vi "Autonomous Independent.vi"   [LabVIEW 2016]
doc: "This VI is called when autonomous begins, and will automatically be terminated when autonomous ends. You can carry out timed or sensor driven robot movement independently without needing to return to the caller."
uses:
  Robot Global Data.vi
  <vilib>/Rock Robotics/Network Tables/NT Read String.vi
  <vilib>/Rock Robotics/WPI/Utilities/WPI_GetSetVariantRefNum.vi
  <vilib>/Rock Robotics/WPI/RobotDrive/WPI_RobotDriveArcadeDrive_Standard(NoSaturation).vi
panel:
  # "Be sure to right-click and choose Data Operations>>Make Current Value default if you want to save the array values with the VI"
types:
  T1 = typedef "WPI_RobotDriveDevRef.ctl" = cluster{"DevStatus":errorcluster, "Motors[]":T2[], "Square Inputs":bool, "Max Output":dbl}
  T2 = typedef "WPI_MotorControlDeviceRef.ctl" = cluster{"DeviceStatus":errorcluster, "Type":T3, "PWM":cluster{"PWM Channel":T4, "DeadBand":T5}, "CAN":cluster{"Device Number":u8, "SetOutput VI Ref":variant, "GetOutput VI Ref":variant, "Enable VI Ref":variant, "Disable VI Ref":variant, "Data":variant}, "Invert":bool}
  T3 = typedef "WPI_MotorControlType.ctl" = enum16{"PWM", "CAN"}
  T4 = typedef "FPGA_DIOPWMChannel.ctl" = enum8{"PWM 0", "PWM 1", "PWM 2", "PWM 3", "PWM 4", "PWM 5", "PWM 6", "PWM 7", "PWM 8", "PWM 9", "PWM MXP 0", "PWM MXP 1", "PWM MXP 2", "PWM MXP 3", "PWM MXP 4", "PWM MXP 5", "PWM MXP 6", "PWM MXP 7", "PWM MXP 8", "PWM MXP 9", "Invalid"}
  T5 = typedef "WPI_PWMDeadband.ctl" = cluster{"Name":string, "maxPositivePwm":i32, "minPositivePwm":i32, "centerPwm":i32, "maxNegativePwm":i32, "minNegativePwm":i32, "angularRange":u16}
  T6 = typedef "WPI_GyroDevRef.ctl" = cluster{"DevStatus":errorcluster, "Analog Channel":T7, "Offset":dbl, "Gain (VoltsPerDegree/Second)":dbl, "Gyro Type":enum16{"Analog", "XRS450"}, "Handle":i32, "SPI Bus":T8, "Device Found":bool, "Sample Rate":dbl, "Calibrate On Open":bool}
  T7 = typedef "FPGA_AIChannel.ctl" = enum8{"AI 0", "AI 1", "AI 2", "AI 3", "AI MXP 0", "AI MXP 1", "AI MXP 2", "AI MXP 3", "Invalid"}
  T8 = typedef "spi_bus.ctl" = enum16{"SPI On-Board, CS0", "SPI On-Board, CS1", "SPI On-Board, CS2", "SPI On-Board, CS3", "SPI MXP", "Invalid"}
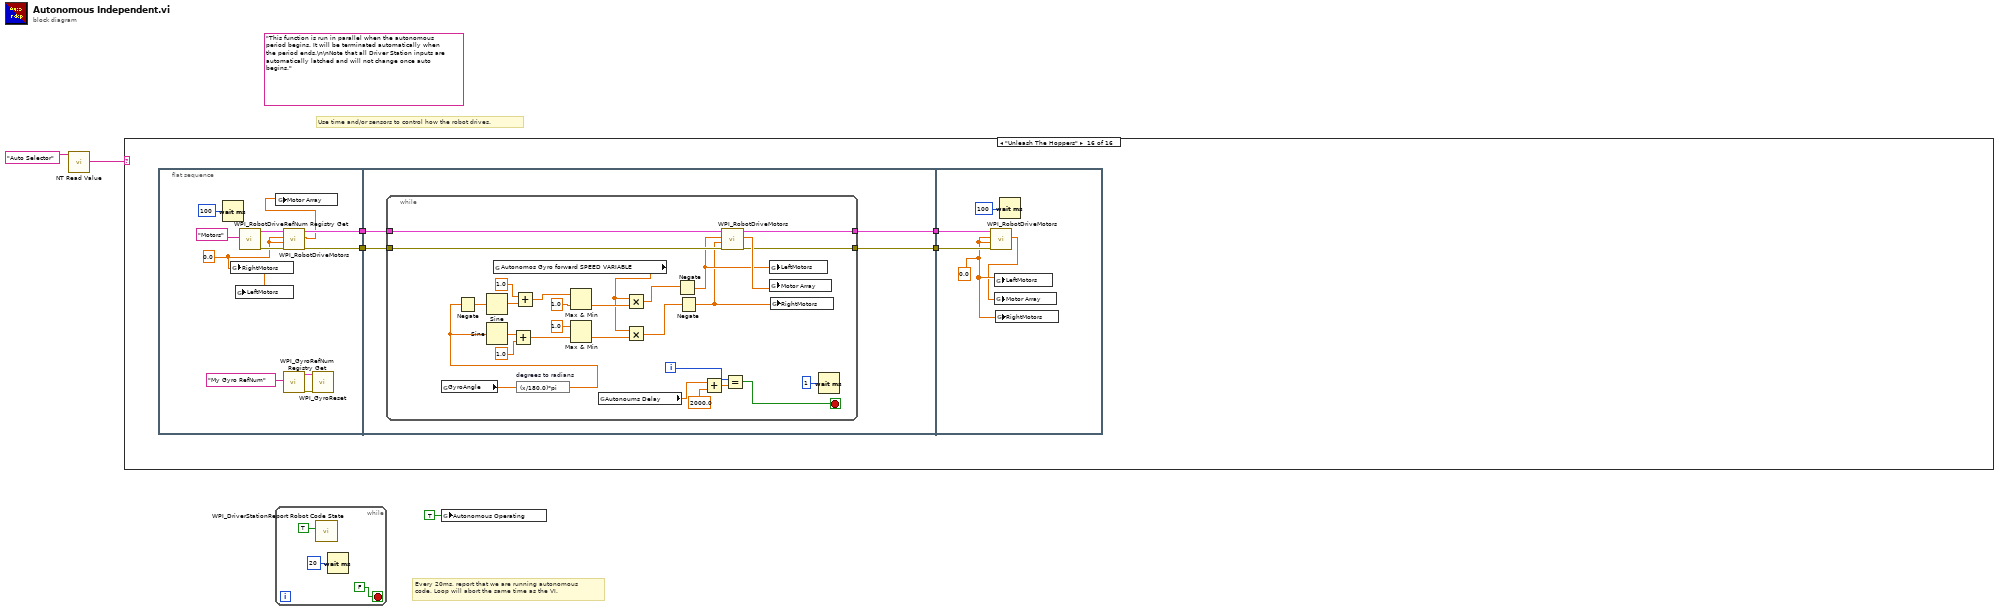
[diagram p0: block diagram]
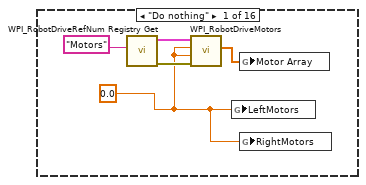
[diagram p2: hidden frame]
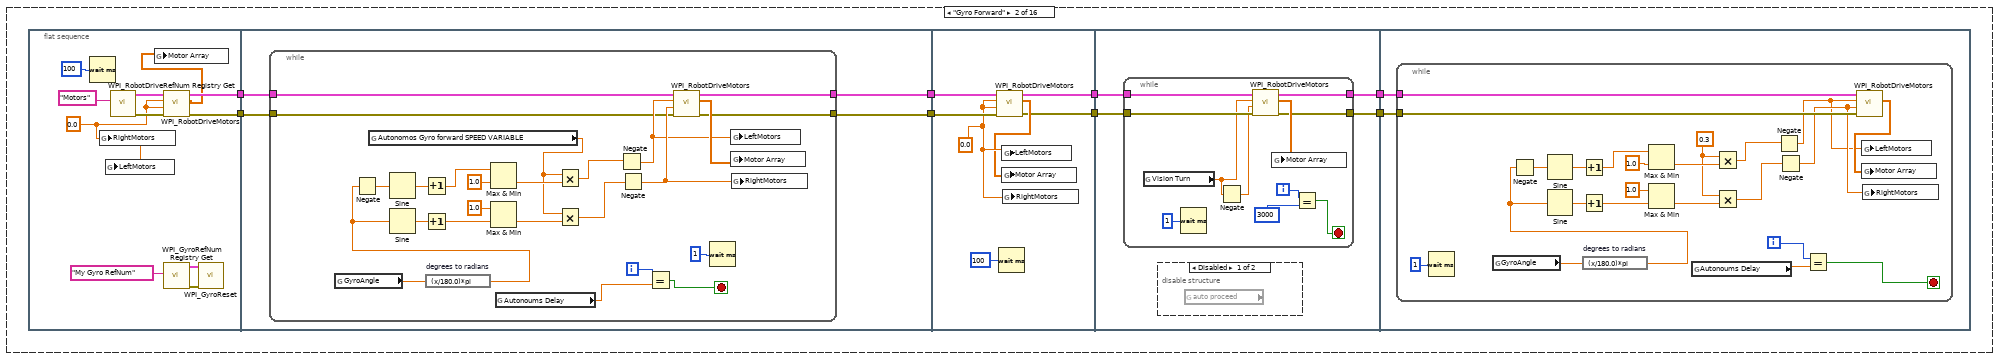
[diagram p3: hidden frame]
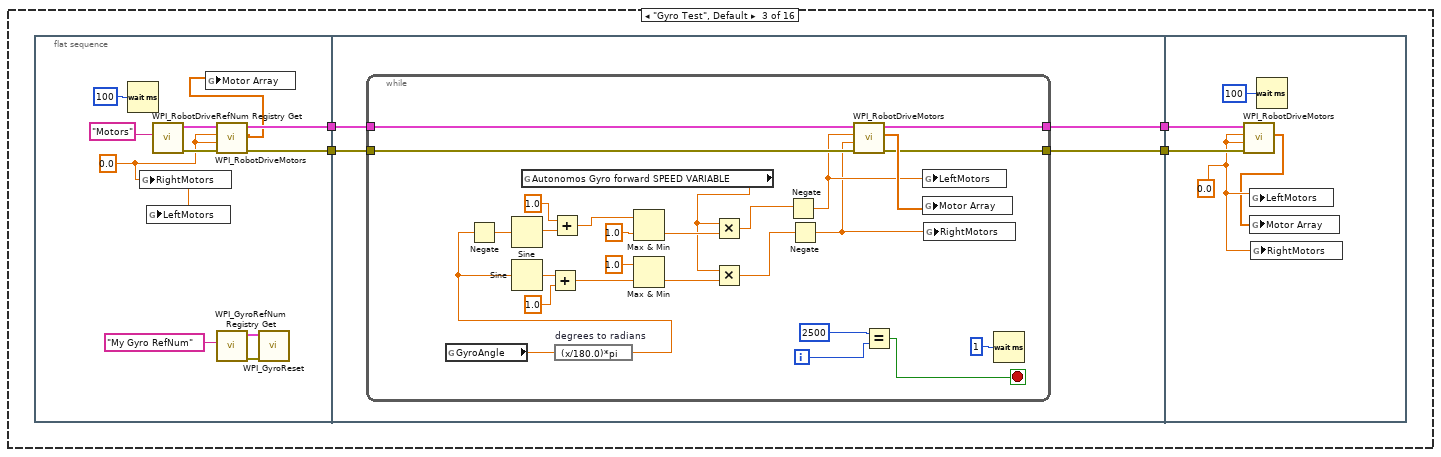
[diagram p5: hidden frame]
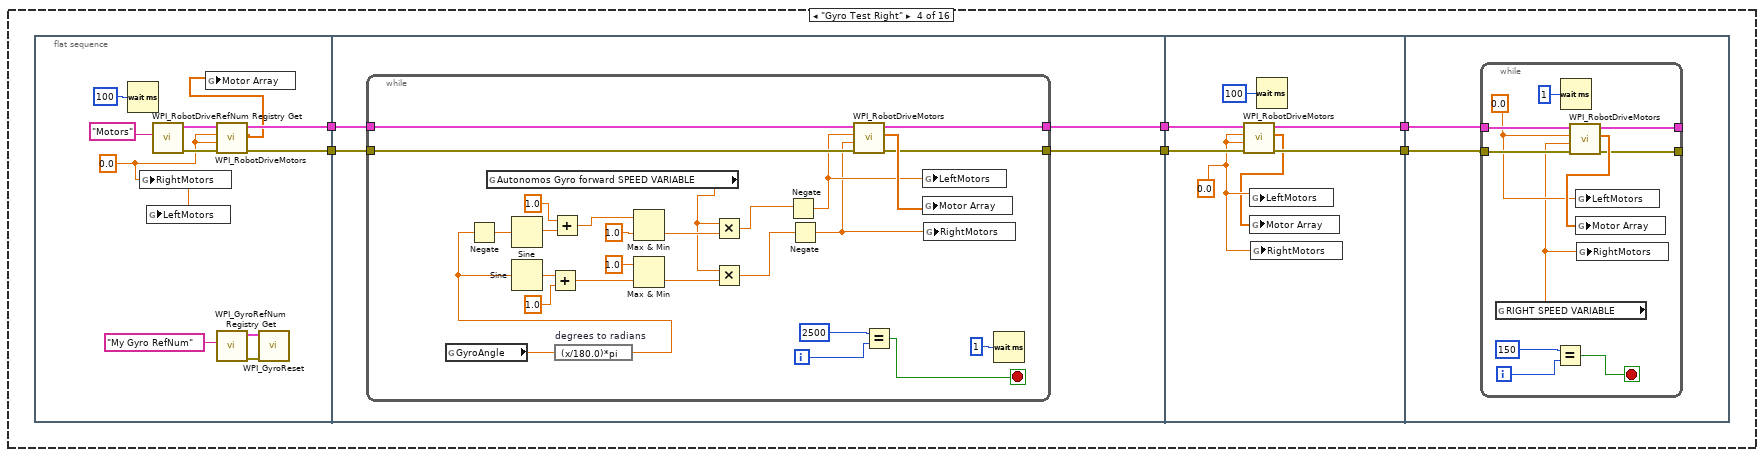
[diagram p6: hidden frame]
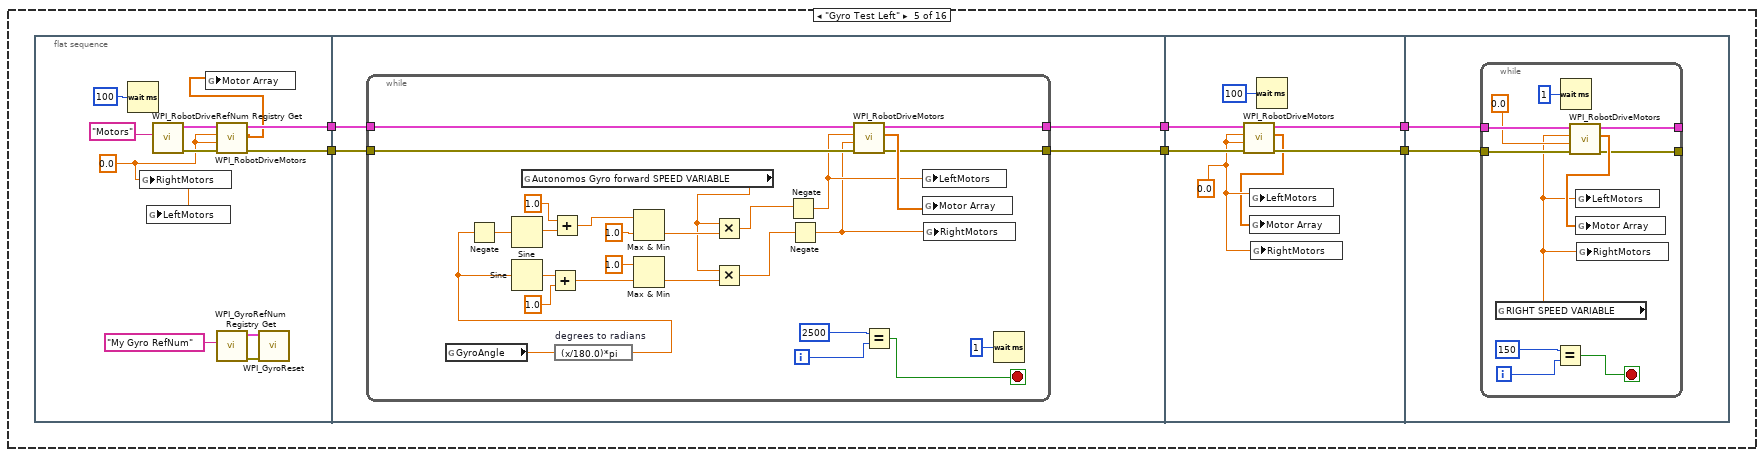
[diagram p7: hidden frame]
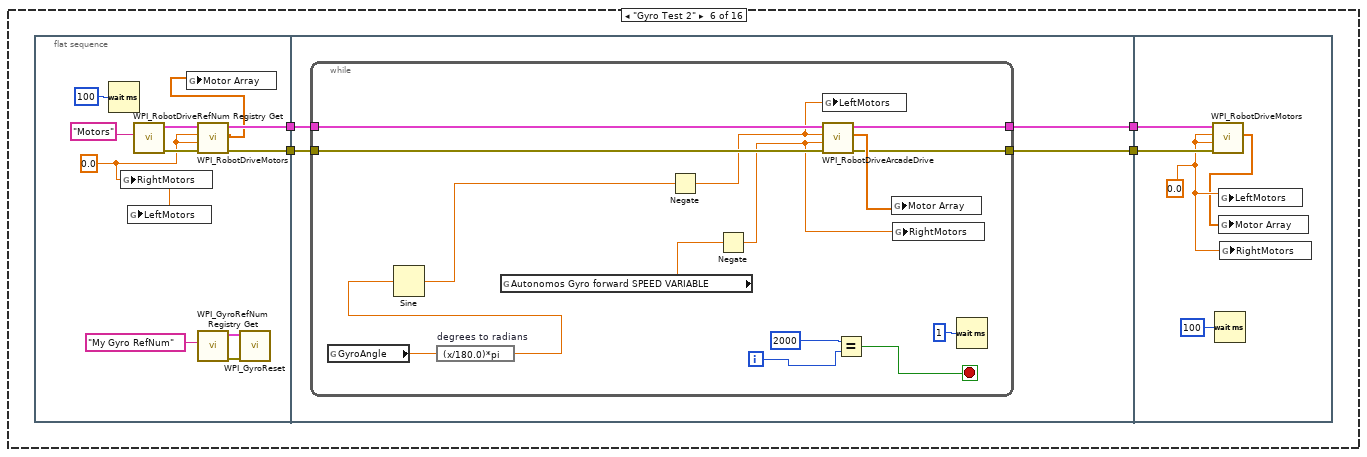
[diagram p8: hidden frame]
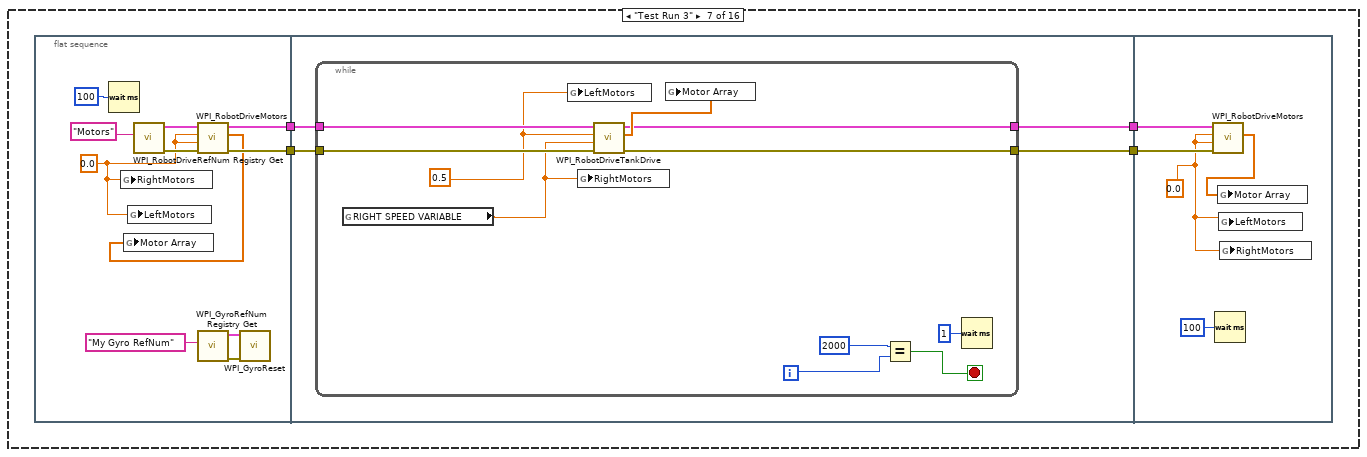
[diagram p9: hidden frame]
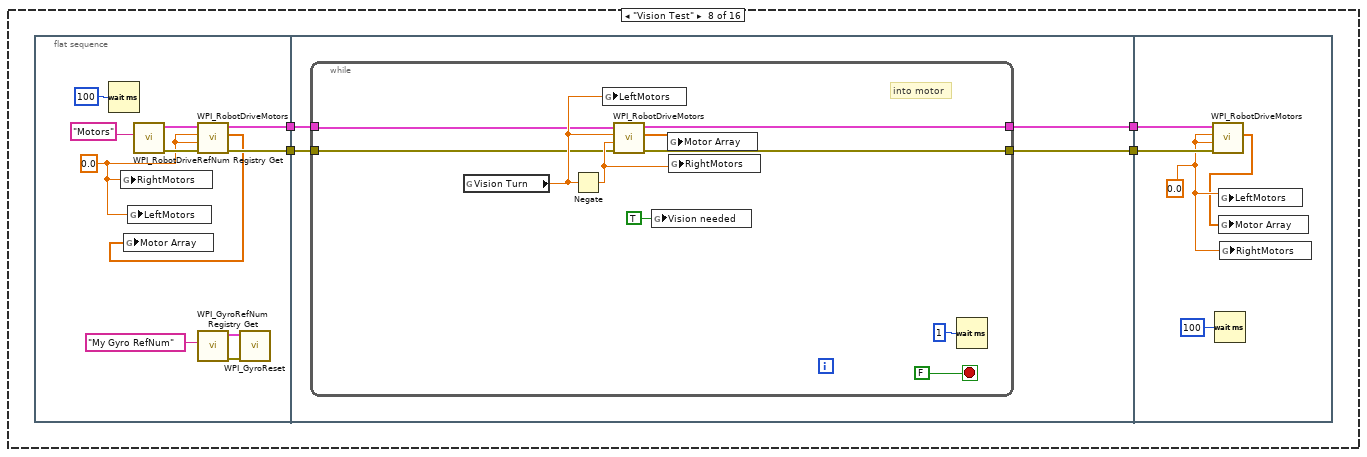
[diagram p10: hidden frame]
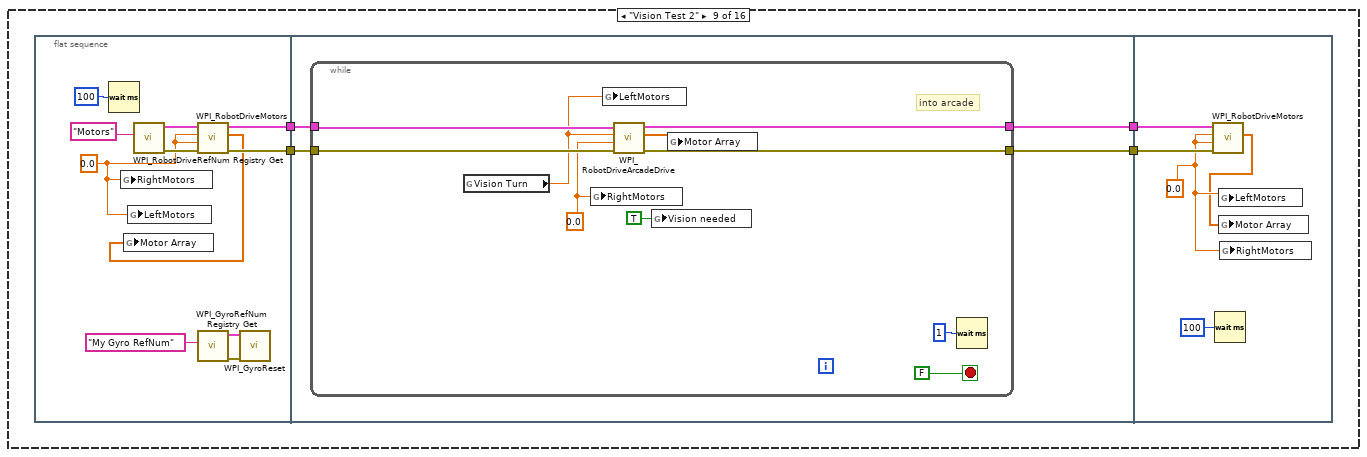
[diagram p11: hidden frame]
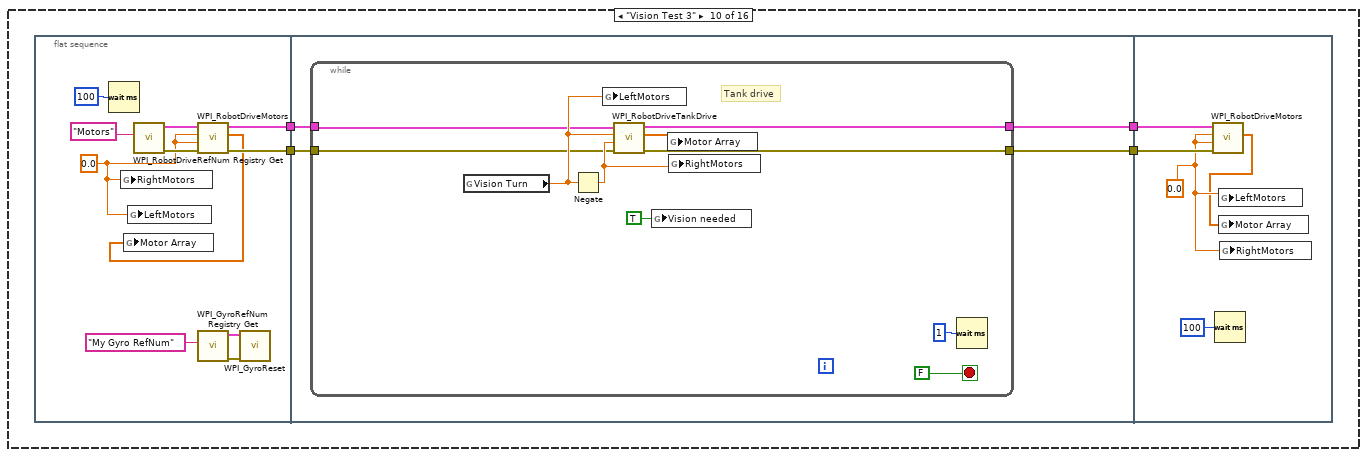
[diagram p12: hidden frame]
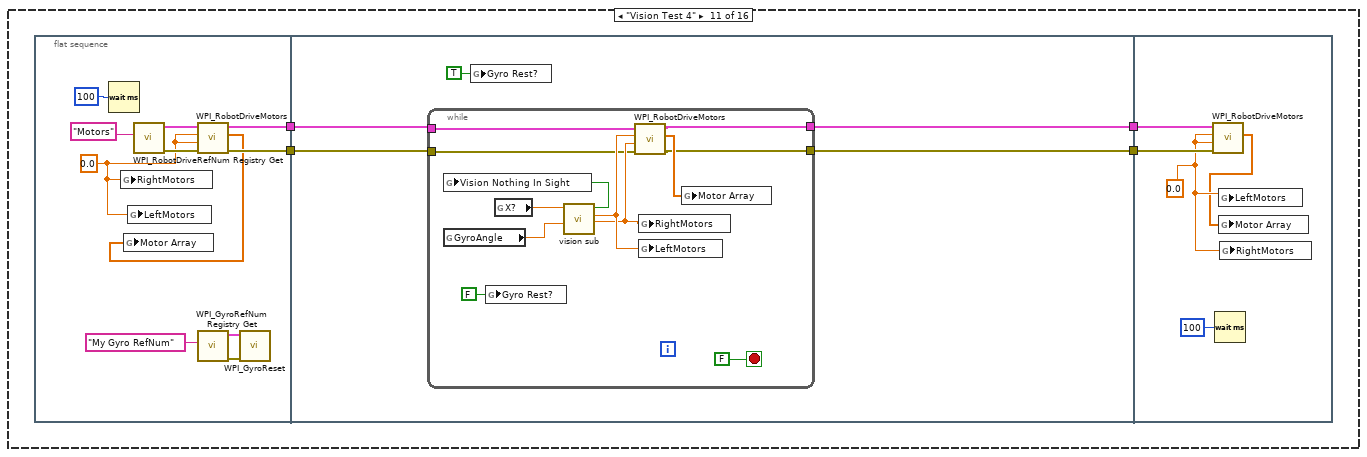
[diagram p13: hidden frame]
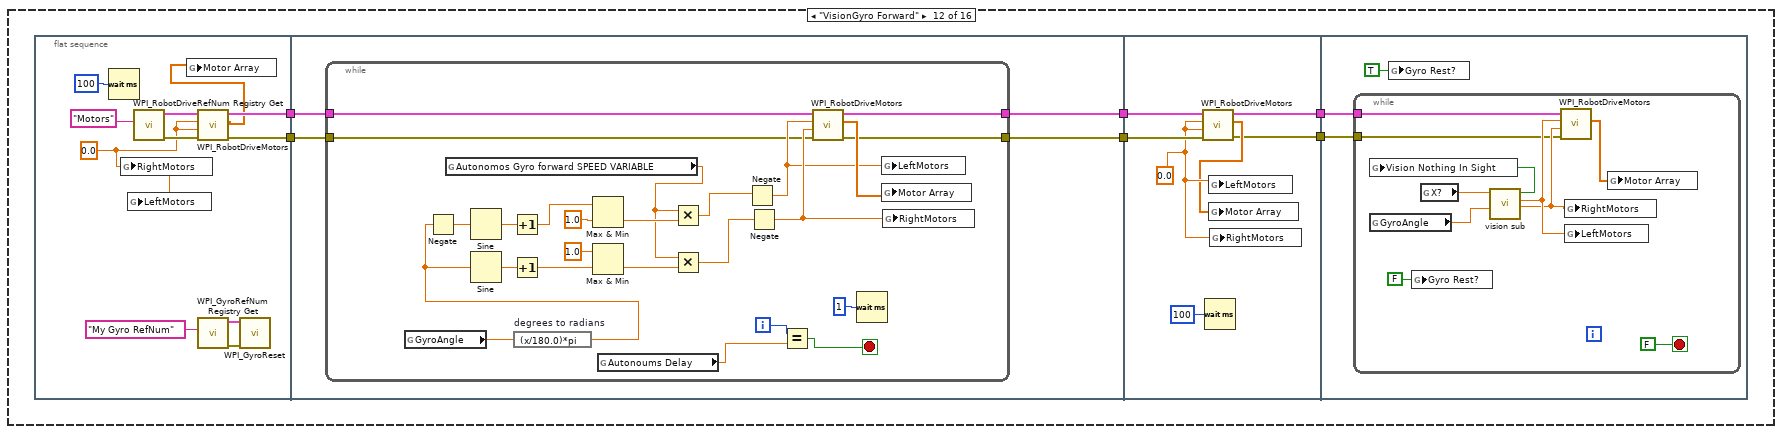
[diagram p14: hidden frame]
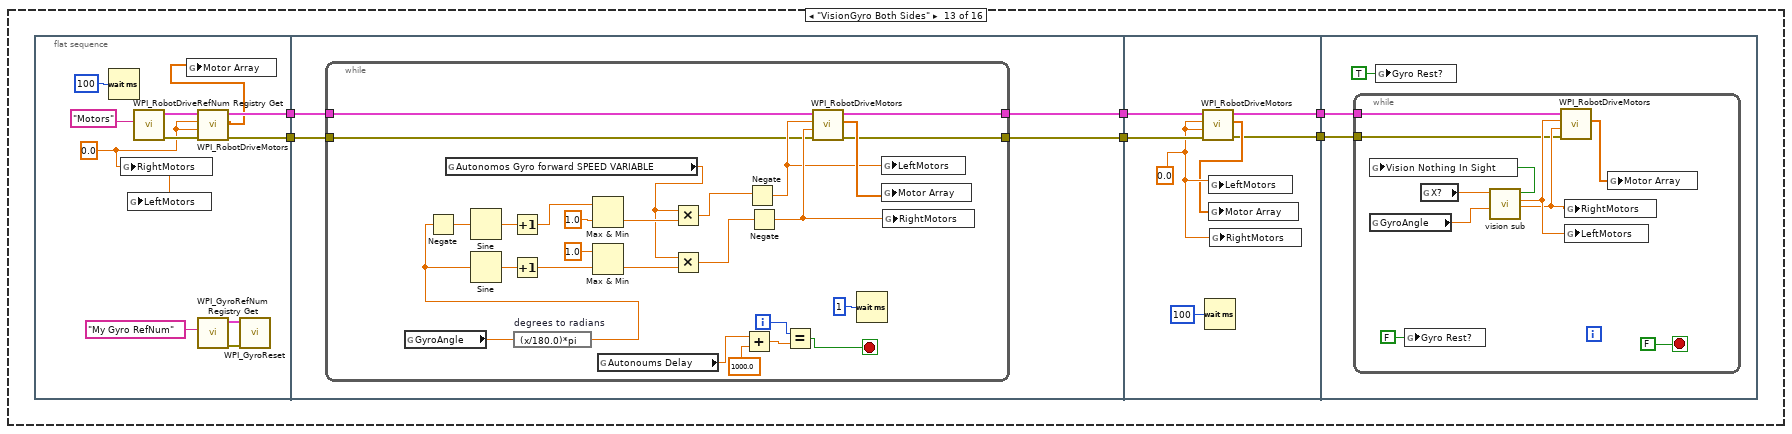
[diagram p15: hidden frame]
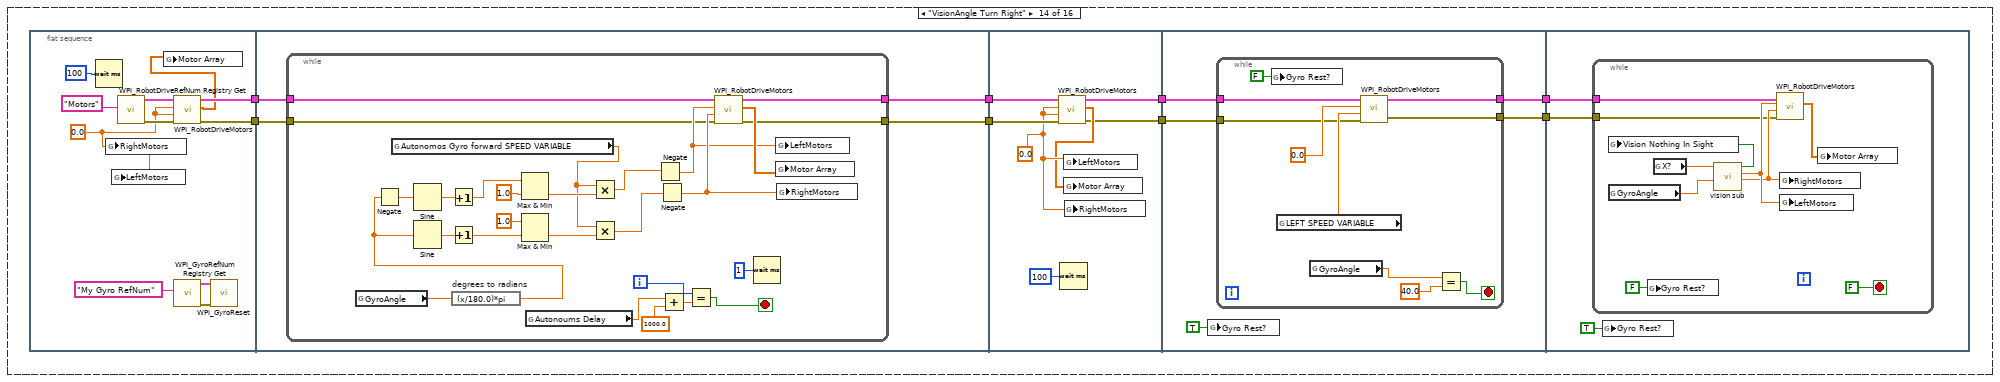
[diagram p16: hidden frame]
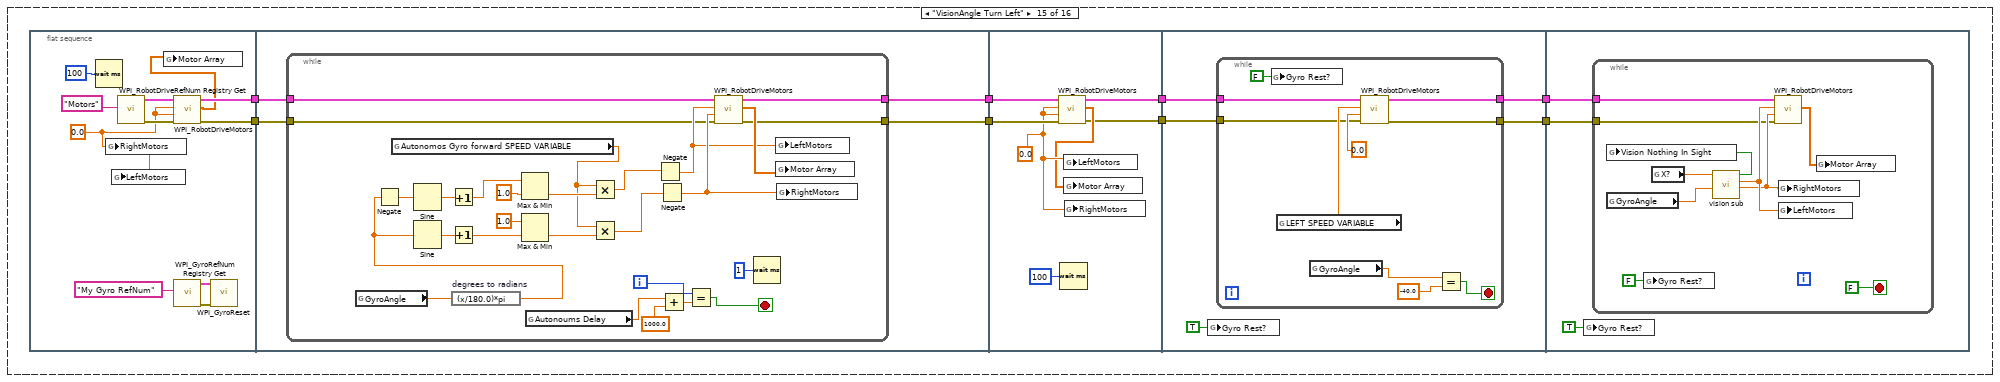
[diagram p17: hidden frame]
diagram:
  (unwired) "This function is run in parallel when the autonomous period begins. It will be terminated automatically when the period ends.\n\nNote that all Driver Station inputs are automatically latched and will not change once auto begins."
  # "Every 20ms, report that we are running autonomous\ncode. Loop will abort the same time as the VI."
  # "Use time and/or sensors to control how the robot drives."
  n1 = call-poly <vilib>:"NT Read Value.vi"("Name"="Auto Selector") -> ("String"=w1:string)  [unwired: 9 in, 1 out]
  n2 = case shown="\"Unleash The Hoppers\"" w1 {
    frame "Do nothing" {
      w5 = 0.0 ("TopLeftMotor")
      n3 = call <vilib>:"WPI_RobotDriveRefNum Registry Get.vi"("refnum name"="Motors") -> ("error out"=w8:errorcluster, "RobotDriveDevRef"=w7:T1)  [unwired: 9 in]
      n4 = call <vilib>:"WPI_RobotDriveMotors.vi"("error in (no error)"=w8, "RightSpeed"=w5, "LeftSpeed"=w5, "RobotDriveDevRef"=w7) -> ("Motor Values"=w4:dbl[])  [unwired: 5 in, 2 out]
      n5 = global write "Robot Global Data.vi" "LeftMotors"(w5) -> ()
      n6 = global write "Robot Global Data.vi" "Motor Array"(w4) -> ()
      n7 = global write "Robot Global Data.vi" "RightMotors"(w5) -> ()
    }
    frame "Gyro Forward" {
      n8 = flat-sequence {
        tunnel: [w21] -> w16
        tunnel: [w19] -> w15
        tunnel: w16 -> [w30]
        tunnel: w15 -> [w29]
        tunnel: [w28] -> w14
        tunnel: [w27] -> w13
        tunnel: w14 -> [w62]
        tunnel: w13 -> [w61]
        tunnel: [w57] -> w12
        tunnel: [w56] -> w11
        tunnel: w12 -> [w66]
        tunnel: w11 -> [w65]
        tunnel: [w64] -> w10
        tunnel: [w63] -> w9
        tunnel: w10 -> [w79]
        tunnel: w9 -> [w78]
        frame #0 {
          w18 = 0.0 ("TopLeftMotor")
          n9 = Wait (ms)(milliseconds to wait=u32 100) -> ()  [unwired: 1 out]
          n10 = global write "Robot Global Data.vi" "RightMotors"(w18) -> ()
          n11 = global write "Robot Global Data.vi" "LeftMotors"(w18) -> ()
          n12 = call <vilib>:"WPI_RobotDriveRefNum Registry Get.vi"("refnum name"="Motors") -> ("error out"=w21:errorcluster, "RobotDriveDevRef"=w20:T1)  [unwired: 9 in]
          n13 = call <vilib>:"WPI_RobotDriveMotors.vi"("RightSpeed"=w18, "LeftSpeed"=w18, "RobotDriveDevRef"=w20) -> ("Motor Values"=w17:dbl[], "RobotDriveDevRef"=w19:T1)  [unwired: 6 in, 1 out]
          n14 = global write "Robot Global Data.vi" "Motor Array"(w17) -> ()
          n15 = call <vilib>:"WPI_GyroRefNum Registry Get.vi"("refnum name"="My Gyro RefNum") -> ("error out"=w24:errorcluster, "GyroDevRef"=w25:T6)  [unwired: 9 in]
          n16 = call <vilib>:"WPI_GyroReset.vi"("error in"=w24, "GyroDevRef"=w25) -> ()  [unwired: 8 in, 2 out]
        }
        frame #1 {
          n17 = while {
            tunnel: w30 -> [w50]
            tunnel: w29 -> [w51]
            tunnel: [w49] -> w28
            tunnel: [w48] -> w27
            i -> [w34]
            stop <- w33 stop-if-true
            n18 = global read "Robot Global Data.vi" "GyroAngle"() -> (w36:dbl)
            n19 = global read "Robot Global Data.vi" "Autonomos Gyro forward SPEED VARIABLE"() -> (w32:dbl)
            n20 = expression code="(x/180.0)*pi" "degrees to radians"(w36) -> (w35:dbl)
            n21 = Negate(x=w35) -> (-x=w41:dbl)
            n22 = Sine(x=w41) -> (sin(x)=w43:dbl)
            n23 = Sine(x=w35) -> (sin(x)=w45:dbl)
            n24 = Increment(x=w43) -> (x+1=w42:dbl)
            n25 = Increment(x=w45) -> (x+1=w44:dbl)
            n26 = Max & Min(x=w42, y=1.0) -> (min(x,y)=w39:dbl)  [unwired: 1 out]
            n27 = Max & Min(x=1.0, y=w44) -> (min(x,y)=w40:dbl)  [unwired: 1 out]
            n28 = global read "Robot Global Data.vi" "Autonoums Delay"() -> (w31:dbl)
            n29 = Multiply(x=w32, y=w39) -> (x*y=w38:dbl)
            n30 = Multiply(x=w32, y=w40) -> (x*y=w37:dbl)
            n31 = Negate(x=w38) -> (-x=w52:dbl)
            n32 = Negate(x=w37) -> (-x=w53:dbl)
            n33 = Equal?(x=w34, y=w31) -> (x = y?=w33:bool)
            n34 = call <vilib>:"WPI_RobotDriveMotors.vi"("error in (no error)"=w50, "RightSpeed"=w53, "LeftSpeed"=w52, "RobotDriveDevRef"=w51) -> ("error out"=w48:errorcluster, "Motor Values"=w54:dbl[], "RobotDriveDevRef"=w49:T1)  [unwired: 5 in]
            n35 = Wait (ms)(milliseconds to wait=u32 1) -> ()  [unwired: 1 out]
            n36 = global write "Robot Global Data.vi" "LeftMotors"(w52) -> ()
            n37 = global write "Robot Global Data.vi" "Motor Array"(w54) -> ()
            n38 = global write "Robot Global Data.vi" "RightMotors"(w53) -> ()
          }
        }
        frame #2 {
          w59 = 0.0 ("LeftSpeed")
          n39 = call <vilib>:"WPI_RobotDriveMotors.vi"("error in (no error)"=w61, "RightSpeed"=w59, "LeftSpeed"=w59, "RobotDriveDevRef"=w62) -> ("error out"=w56:errorcluster, "Motor Values"=w58:dbl[], "RobotDriveDevRef"=w57:T1)  [unwired: 5 in]
          n40 = Wait (ms)(milliseconds to wait=u32 100) -> ()  [unwired: 1 out]
          n41 = global write "Robot Global Data.vi" "LeftMotors"(w59) -> ()
          n42 = global write "Robot Global Data.vi" "Motor Array"(w58) -> ()
          n43 = global write "Robot Global Data.vi" "RightMotors"(w59) -> ()
        }
        frame #3 {
          n44 = while {
            tunnel: w66 -> [w75]
            tunnel: w65 -> [w74]
            tunnel: [w73] -> w64
            tunnel: [w72] -> w63
            i -> [w70]
            stop <- w69 stop-if-true
            n45 = global read "Robot Global Data.vi" "Vision Turn"() -> (w67:dbl)
            n46 = Wait (ms)(milliseconds to wait=u32 1) -> ()  [unwired: 1 out]
            n47 = Negate(x=w67) -> (-x=w68:dbl)
            n48 = call <vilib>:"WPI_RobotDriveMotors.vi"("error in (no error)"=w74, "RightSpeed"=w68, "LeftSpeed"=w67, "RobotDriveDevRef"=w75) -> ("error out"=w72:errorcluster, "Motor Values"=w77:dbl[], "RobotDriveDevRef"=w73:T1)  [unwired: 5 out]
            n49 = global write "Robot Global Data.vi" "Motor Array"(w77) -> ()
            n50 = Equal?(x=w70, y=u32 3000 ("milliseconds to wait")) -> (x = y?=w69:bool)
          }
          n51 = disable-structure shown="Disabled" {
            frame Disabled {
              n52 = global read "Robot Global Data.vi" "auto proceed"() -> ()  [unwired: 1 out]
            }
            frame Enabled {
            }
          }
        }
        frame #4 {
          n53 = while {
            tunnel: w79 -> [w101]
            tunnel: w78 -> [w100]
            i -> [w82]
            stop <- w81 stop-if-true
            w87 = 0.3
            n54 = Wait (ms)(milliseconds to wait=u32 1) -> ()  [unwired: 1 out]
            n55 = global read "Robot Global Data.vi" "GyroAngle"() -> (w86:dbl)
            n56 = expression code="(x/180.0)*pi" "degrees to radians"(w86) -> (w85:dbl)
            n57 = Negate(x=w85) -> (-x=w92:dbl)
            n58 = Sine(x=w92) -> (sin(x)=w94:dbl)
            n59 = Sine(x=w85) -> (sin(x)=w96:dbl)
            n60 = Increment(x=w94) -> (x+1=w93:dbl)
            n61 = Increment(x=w96) -> (x+1=w95:dbl)
            n62 = Max & Min(x=w93, y=1.0) -> (min(x,y)=w90:dbl)  [unwired: 1 out]
            n63 = Max & Min(x=1.0, y=w95) -> (min(x,y)=w91:dbl)  [unwired: 1 out]
            n64 = global read "Robot Global Data.vi" "Autonoums Delay"() -> (w80:dbl)
            n65 = Multiply(x=w87, y=w90) -> (x*y=w89:dbl)
            n66 = Multiply(x=w87, y=w91) -> (x*y=w88:dbl)
            n67 = Negate(x=w89) -> (-x=w83:dbl)
            n68 = Negate(x=w88) -> (-x=w84:dbl)
            n69 = Equal?(x=w82, y=w80) -> (x = y?=w81:bool)
            n70 = call <vilib>:"WPI_RobotDriveMotors.vi"("error in (no error)"=w100, "RightSpeed"=w84, "LeftSpeed"=w83, "RobotDriveDevRef"=w101) -> ("Motor Values"=w102:dbl[])  [unwired: 5 in, 2 out]
            n71 = global write "Robot Global Data.vi" "LeftMotors"(w83) -> ()
            n72 = global write "Robot Global Data.vi" "Motor Array"(w102) -> ()
            n73 = global write "Robot Global Data.vi" "RightMotors"(w84) -> ()
          }
        }
      }
    }
    frame "Gyro Test", Default {
      n74 = flat-sequence {
        tunnel: [w116] -> w106
        tunnel: [w115] -> w105
        tunnel: w106 -> [w120]
        tunnel: w105 -> [w119]
        tunnel: [w118] -> w104
        tunnel: [w117] -> w103
        tunnel: w104 -> [w152]
        tunnel: w103 -> [w151]
        frame #0 {
          w108 = 0.0 ("TopLeftMotor")
          n75 = Wait (ms)(milliseconds to wait=u32 100) -> ()  [unwired: 1 out]
          n76 = global write "Robot Global Data.vi" "RightMotors"(w108) -> ()
          n77 = global write "Robot Global Data.vi" "LeftMotors"(w108) -> ()
          n78 = call <vilib>:"WPI_RobotDriveRefNum Registry Get.vi"("refnum name"="Motors") -> ("error out"=w116:errorcluster, "RobotDriveDevRef"=w109:T1)  [unwired: 9 in]
          n79 = call <vilib>:"WPI_RobotDriveMotors.vi"("RightSpeed"=w108, "LeftSpeed"=w108, "RobotDriveDevRef"=w109) -> ("Motor Values"=w107:dbl[], "RobotDriveDevRef"=w115:T1)  [unwired: 6 in, 1 out]
          n80 = global write "Robot Global Data.vi" "Motor Array"(w107) -> ()
          n81 = call <vilib>:"WPI_GyroRefNum Registry Get.vi"("refnum name"="My Gyro RefNum") -> ("error out"=w112:errorcluster, "GyroDevRef"=w113:T6)  [unwired: 9 in]
          n82 = call <vilib>:"WPI_GyroReset.vi"("error in"=w112, "GyroDevRef"=w113) -> ()  [unwired: 8 in, 2 out]
        }
        frame #1 {
          n83 = while {
            tunnel: w120 -> [w144]
            tunnel: w119 -> [w145]
            tunnel: [w143] -> w118
            tunnel: [w142] -> w117
            i -> [w123]
            stop <- w122 stop-if-true
            n84 = global read "Robot Global Data.vi" "GyroAngle"() -> (w134:dbl)
            n85 = global read "Robot Global Data.vi" "Autonomos Gyro forward SPEED VARIABLE"() -> (w121:dbl)
            n86 = expression code="(x/180.0)*pi" "degrees to radians"(w134) -> (w133:dbl)
            n87 = Negate(x=w133) -> (-x=w139:dbl)
            n88 = Sine(x=w139) -> (sin(x)=w128:dbl)
            n89 = Sine(x=w133) -> (sin(x)=w130:dbl)
            n90 = Add(x=w130, y=1.0 ("x")) -> (x+y=w129:dbl)
            n91 = Add(x=1.0, y=w128) -> (x+y=w127:dbl)
            n92 = Max & Min(x=w127, y=1.0) -> (min(x,y)=w137:dbl)  [unwired: 1 out]
            n93 = Max & Min(x=1.0, y=w129) -> (min(x,y)=w138:dbl)  [unwired: 1 out]
            n94 = Multiply(x=w121, y=w137) -> (x*y=w136:dbl)
            n95 = Multiply(x=w121, y=w138) -> (x*y=w135:dbl)
            n96 = Negate(x=w136) -> (-x=w126:dbl)
            n97 = Negate(x=w135) -> (-x=w125:dbl)
            n98 = call <vilib>:"WPI_RobotDriveMotors.vi"("error in (no error)"=w144, "RightSpeed"=w125, "LeftSpeed"=w126, "RobotDriveDevRef"=w145) -> ("error out"=w142:errorcluster, "Motor Values"=w146:dbl[], "RobotDriveDevRef"=w143:T1)  [unwired: 5 in]
            n99 = Equal?(x=2500, y=w123) -> (x = y?=w122:bool)
            n100 = global write "Robot Global Data.vi" "LeftMotors"(w126) -> ()
            n101 = global write "Robot Global Data.vi" "Motor Array"(w146) -> ()
            n102 = global write "Robot Global Data.vi" "RightMotors"(w125) -> ()
            n103 = Wait (ms)(milliseconds to wait=u32 1) -> ()  [unwired: 1 out]
          }
        }
        frame #2 {
          w149 = 0.0 ("LeftSpeed")
          n104 = call <vilib>:"WPI_RobotDriveMotors.vi"("error in (no error)"=w151, "RightSpeed"=w149, "LeftSpeed"=w149, "RobotDriveDevRef"=w152) -> ("Motor Values"=w148:dbl[])  [unwired: 5 in, 2 out]
          n105 = global write "Robot Global Data.vi" "LeftMotors"(w149) -> ()
          n106 = global write "Robot Global Data.vi" "Motor Array"(w148) -> ()
          n107 = global write "Robot Global Data.vi" "RightMotors"(w149) -> ()
          n108 = Wait (ms)(milliseconds to wait=u32 100) -> ()  [unwired: 1 out]
        }
      }
    }
    frame "Gyro Test Right" {
      n109 = flat-sequence {
        tunnel: [w168] -> w158
        tunnel: [w167] -> w157
        tunnel: w158 -> [w172]
        tunnel: w157 -> [w171]
        tunnel: [w170] -> w156
        tunnel: [w169] -> w155
        tunnel: w156 -> [w206]
        tunnel: w155 -> [w205]
        tunnel: [w204] -> w154
        tunnel: [w203] -> w153
        tunnel: w154 -> [w208]
        tunnel: w153 -> [w207]
        frame #0 {
          w160 = 0.0 ("TopLeftMotor")
          n110 = Wait (ms)(milliseconds to wait=u32 100) -> ()  [unwired: 1 out]
          n111 = global write "Robot Global Data.vi" "RightMotors"(w160) -> ()
          n112 = global write "Robot Global Data.vi" "LeftMotors"(w160) -> ()
          n113 = call <vilib>:"WPI_RobotDriveRefNum Registry Get.vi"("refnum name"="Motors") -> ("error out"=w168:errorcluster, "RobotDriveDevRef"=w161:T1)  [unwired: 9 in]
          n114 = call <vilib>:"WPI_RobotDriveMotors.vi"("RightSpeed"=w160, "LeftSpeed"=w160, "RobotDriveDevRef"=w161) -> ("Motor Values"=w159:dbl[], "RobotDriveDevRef"=w167:T1)  [unwired: 6 in, 1 out]
          n115 = global write "Robot Global Data.vi" "Motor Array"(w159) -> ()
          n116 = call <vilib>:"WPI_GyroRefNum Registry Get.vi"("refnum name"="My Gyro RefNum") -> ("error out"=w164:errorcluster, "GyroDevRef"=w165:T6)  [unwired: 9 in]
          n117 = call <vilib>:"WPI_GyroReset.vi"("error in"=w164, "GyroDevRef"=w165) -> ()  [unwired: 8 in, 2 out]
        }
        frame #1 {
          n118 = while {
            tunnel: w172 -> [w196]
            tunnel: w171 -> [w197]
            tunnel: [w195] -> w170
            tunnel: [w194] -> w169
            i -> [w175]
            stop <- w174 stop-if-true
            n119 = global read "Robot Global Data.vi" "GyroAngle"() -> (w186:dbl)
            n120 = global read "Robot Global Data.vi" "Autonomos Gyro forward SPEED VARIABLE"() -> (w173:dbl)
            n121 = expression code="(x/180.0)*pi" "degrees to radians"(w186) -> (w185:dbl)
            n122 = Negate(x=w185) -> (-x=w191:dbl)
            n123 = Sine(x=w191) -> (sin(x)=w180:dbl)
            n124 = Sine(x=w185) -> (sin(x)=w182:dbl)
            n125 = Add(x=w182, y=1.0 ("x")) -> (x+y=w181:dbl)
            n126 = Add(x=1.0, y=w180) -> (x+y=w179:dbl)
            n127 = Max & Min(x=w179, y=1.0) -> (min(x,y)=w189:dbl)  [unwired: 1 out]
            n128 = Max & Min(x=1.0, y=w181) -> (min(x,y)=w190:dbl)  [unwired: 1 out]
            n129 = Multiply(x=w173, y=w189) -> (x*y=w188:dbl)
            n130 = Multiply(x=w173, y=w190) -> (x*y=w187:dbl)
            n131 = Negate(x=w188) -> (-x=w178:dbl)
            n132 = Negate(x=w187) -> (-x=w177:dbl)
            n133 = call <vilib>:"WPI_RobotDriveMotors.vi"("error in (no error)"=w196, "RightSpeed"=w177, "LeftSpeed"=w178, "RobotDriveDevRef"=w197) -> ("error out"=w194:errorcluster, "Motor Values"=w198:dbl[], "RobotDriveDevRef"=w195:T1)  [unwired: 5 in]
            n134 = Equal?(x=2500, y=w175) -> (x = y?=w174:bool)
            n135 = global write "Robot Global Data.vi" "LeftMotors"(w178) -> ()
            n136 = global write "Robot Global Data.vi" "Motor Array"(w198) -> ()
            n137 = global write "Robot Global Data.vi" "RightMotors"(w177) -> ()
            n138 = Wait (ms)(milliseconds to wait=u32 1) -> ()  [unwired: 1 out]
          }
        }
        frame #2 {
          w201 = 0.0 ("LeftSpeed")
          n139 = call <vilib>:"WPI_RobotDriveMotors.vi"("error in (no error)"=w205, "RightSpeed"=w201, "LeftSpeed"=w201, "RobotDriveDevRef"=w206) -> ("error out"=w203:errorcluster, "Motor Values"=w200:dbl[], "RobotDriveDevRef"=w204:T1)  [unwired: 5 in]
          n140 = global write "Robot Global Data.vi" "LeftMotors"(w201) -> ()
          n141 = global write "Robot Global Data.vi" "Motor Array"(w200) -> ()
          n142 = global write "Robot Global Data.vi" "RightMotors"(w201) -> ()
          n143 = Wait (ms)(milliseconds to wait=u32 100) -> ()  [unwired: 1 out]
        }
        frame #3 {
          n144 = while {
            tunnel: w208 -> [w219]
            tunnel: w207 -> [w218]
            tunnel: [w212] -> _
            tunnel: [w211] -> _
            i -> [w215]
            stop <- w213 stop-if-true
            w210 = 0.0 ("LeftSpeed")
            n145 = global read "Robot Global Data.vi" "RIGHT SPEED VARIABLE"() -> (w209:dbl)
            n146 = Equal?(x=150, y=w215) -> (x = y?=w213:bool)
            n147 = Wait (ms)(milliseconds to wait=u32 1) -> ()  [unwired: 1 out]
            n148 = call <vilib>:"WPI_RobotDriveMotors.vi"("error in (no error)"=w218, "RightSpeed"=w209, "LeftSpeed"=w210, "RobotDriveDevRef"=w219) -> ("error out"=w211:errorcluster, "Motor Values"=w216:dbl[], "RobotDriveDevRef"=w212:T1)  [unwired: 5 in]
            n149 = global write "Robot Global Data.vi" "LeftMotors"(w210) -> ()
            n150 = global write "Robot Global Data.vi" "Motor Array"(w216) -> ()
            n151 = global write "Robot Global Data.vi" "RightMotors"(w209) -> ()
          }
        }
      }
    }
    frame "Gyro Test Left" {
      n152 = flat-sequence {
        tunnel: [w235] -> w225
        tunnel: [w234] -> w224
        tunnel: w225 -> [w239]
        tunnel: w224 -> [w238]
        tunnel: [w237] -> w223
        tunnel: [w236] -> w222
        tunnel: w223 -> [w273]
        tunnel: w222 -> [w272]
        tunnel: [w271] -> w221
        tunnel: [w270] -> w220
        tunnel: w221 -> [w275]
        tunnel: w220 -> [w274]
        frame #0 {
          w227 = 0.0 ("TopLeftMotor")
          n153 = Wait (ms)(milliseconds to wait=u32 100) -> ()  [unwired: 1 out]
          n154 = global write "Robot Global Data.vi" "RightMotors"(w227) -> ()
          n155 = global write "Robot Global Data.vi" "LeftMotors"(w227) -> ()
          n156 = call <vilib>:"WPI_RobotDriveRefNum Registry Get.vi"("refnum name"="Motors") -> ("error out"=w235:errorcluster, "RobotDriveDevRef"=w228:T1)  [unwired: 9 in]
          n157 = call <vilib>:"WPI_RobotDriveMotors.vi"("RightSpeed"=w227, "LeftSpeed"=w227, "RobotDriveDevRef"=w228) -> ("Motor Values"=w226:dbl[], "RobotDriveDevRef"=w234:T1)  [unwired: 6 in, 1 out]
          n158 = global write "Robot Global Data.vi" "Motor Array"(w226) -> ()
          n159 = call <vilib>:"WPI_GyroRefNum Registry Get.vi"("refnum name"="My Gyro RefNum") -> ("error out"=w231:errorcluster, "GyroDevRef"=w232:T6)  [unwired: 9 in]
          n160 = call <vilib>:"WPI_GyroReset.vi"("error in"=w231, "GyroDevRef"=w232) -> ()  [unwired: 8 in, 2 out]
        }
        frame #1 {
          n161 = while {
            tunnel: w239 -> [w263]
            tunnel: w238 -> [w264]
            tunnel: [w262] -> w237
            tunnel: [w261] -> w236
            i -> [w242]
            stop <- w241 stop-if-true
            n162 = global read "Robot Global Data.vi" "GyroAngle"() -> (w253:dbl)
            n163 = global read "Robot Global Data.vi" "Autonomos Gyro forward SPEED VARIABLE"() -> (w240:dbl)
            n164 = expression code="(x/180.0)*pi" "degrees to radians"(w253) -> (w252:dbl)
            n165 = Negate(x=w252) -> (-x=w258:dbl)
            n166 = Sine(x=w258) -> (sin(x)=w247:dbl)
            n167 = Sine(x=w252) -> (sin(x)=w249:dbl)
            n168 = Add(x=w249, y=1.0 ("x")) -> (x+y=w248:dbl)
            n169 = Add(x=1.0, y=w247) -> (x+y=w246:dbl)
            n170 = Max & Min(x=w246, y=1.0) -> (min(x,y)=w256:dbl)  [unwired: 1 out]
            n171 = Max & Min(x=1.0, y=w248) -> (min(x,y)=w257:dbl)  [unwired: 1 out]
            n172 = Multiply(x=w240, y=w256) -> (x*y=w255:dbl)
            n173 = Multiply(x=w240, y=w257) -> (x*y=w254:dbl)
            n174 = Negate(x=w255) -> (-x=w245:dbl)
            n175 = Negate(x=w254) -> (-x=w244:dbl)
            n176 = call <vilib>:"WPI_RobotDriveMotors.vi"("error in (no error)"=w263, "RightSpeed"=w244, "LeftSpeed"=w245, "RobotDriveDevRef"=w264) -> ("error out"=w261:errorcluster, "Motor Values"=w265:dbl[], "RobotDriveDevRef"=w262:T1)  [unwired: 5 in]
            n177 = Equal?(x=2500, y=w242) -> (x = y?=w241:bool)
            n178 = global write "Robot Global Data.vi" "LeftMotors"(w245) -> ()
            n179 = global write "Robot Global Data.vi" "Motor Array"(w265) -> ()
            n180 = global write "Robot Global Data.vi" "RightMotors"(w244) -> ()
            n181 = Wait (ms)(milliseconds to wait=u32 1) -> ()  [unwired: 1 out]
          }
        }
        frame #2 {
          w268 = 0.0 ("LeftSpeed")
          n182 = call <vilib>:"WPI_RobotDriveMotors.vi"("error in (no error)"=w272, "RightSpeed"=w268, "LeftSpeed"=w268, "RobotDriveDevRef"=w273) -> ("error out"=w270:errorcluster, "Motor Values"=w267:dbl[], "RobotDriveDevRef"=w271:T1)  [unwired: 5 in]
          n183 = global write "Robot Global Data.vi" "LeftMotors"(w268) -> ()
          n184 = global write "Robot Global Data.vi" "Motor Array"(w267) -> ()
          n185 = global write "Robot Global Data.vi" "RightMotors"(w268) -> ()
          n186 = Wait (ms)(milliseconds to wait=u32 100) -> ()  [unwired: 1 out]
        }
        frame #3 {
          n187 = while {
            tunnel: w275 -> [w286]
            tunnel: w274 -> [w285]
            tunnel: [w279] -> _
            tunnel: [w278] -> _
            i -> [w282]
            stop <- w280 stop-if-true
            n188 = global read "Robot Global Data.vi" "RIGHT SPEED VARIABLE"() -> (w276:dbl)
            n189 = Equal?(x=150, y=w282) -> (x = y?=w280:bool)
            n190 = Wait (ms)(milliseconds to wait=u32 1) -> ()  [unwired: 1 out]
            n191 = call <vilib>:"WPI_RobotDriveMotors.vi"("error in (no error)"=w285, "RightSpeed"=0.0 ("LeftSpeed"), "LeftSpeed"=w276, "RobotDriveDevRef"=w286) -> ("error out"=w278:errorcluster, "Motor Values"=w283:dbl[], "RobotDriveDevRef"=w279:T1)  [unwired: 5 in]
            n192 = global write "Robot Global Data.vi" "LeftMotors"(w276) -> ()
            n193 = global write "Robot Global Data.vi" "Motor Array"(w283) -> ()
            n194 = global write "Robot Global Data.vi" "RightMotors"(w276) -> ()
          }
        }
      }
    }
    frame "Gyro Test 2" {
      n195 = flat-sequence {
        tunnel: [w295] -> w290
        tunnel: [w293] -> w289
        tunnel: w290 -> [w304]
        tunnel: w289 -> [w303]
        tunnel: [w302] -> w288
        tunnel: [w301] -> w287
        tunnel: w288 -> [w324]
        tunnel: w287 -> [w323]
        frame #0 {
          w292 = 0.0 ("TopLeftMotor")
          n196 = Wait (ms)(milliseconds to wait=u32 100) -> ()  [unwired: 1 out]
          n197 = global write "Robot Global Data.vi" "RightMotors"(w292) -> ()
          n198 = global write "Robot Global Data.vi" "LeftMotors"(w292) -> ()
          n199 = call <vilib>:"WPI_RobotDriveRefNum Registry Get.vi"("refnum name"="Motors") -> ("error out"=w295:errorcluster, "RobotDriveDevRef"=w294:T1)  [unwired: 9 in]
          n200 = call <vilib>:"WPI_RobotDriveMotors.vi"("RightSpeed"=w292, "LeftSpeed"=w292, "RobotDriveDevRef"=w294) -> ("Motor Values"=w291:dbl[], "RobotDriveDevRef"=w293:T1)  [unwired: 6 in, 1 out]
          n201 = global write "Robot Global Data.vi" "Motor Array"(w291) -> ()
          n202 = call <vilib>:"WPI_GyroRefNum Registry Get.vi"("refnum name"="My Gyro RefNum") -> ("error out"=w298:errorcluster, "GyroDevRef"=w299:T6)  [unwired: 9 in]
          n203 = call <vilib>:"WPI_GyroReset.vi"("error in"=w298, "GyroDevRef"=w299) -> ()  [unwired: 8 in, 2 out]
        }
        frame #1 {
          n204 = while {
            tunnel: w304 -> [w316]
            tunnel: w303 -> [w317]
            tunnel: [w315] -> w302
            tunnel: [w314] -> w301
            i -> [w308]
            stop <- w306 stop-if-true
            n205 = global read "Robot Global Data.vi" "GyroAngle"() -> (w312:dbl)
            n206 = expression code="(x/180.0)*pi" "degrees to radians"(w312) -> (w313:dbl)
            n207 = Sine(x=w313) -> (sin(x)=w307:dbl)
            n208 = global read "Robot Global Data.vi" "Autonomos Gyro forward SPEED VARIABLE"() -> (w305:dbl)
            n209 = Negate(x=w307) -> (-x=w311:dbl)
            n210 = Negate(x=w305) -> (-x=w310:dbl)
            n211 = global write "Robot Global Data.vi" "LeftMotors"(w311) -> ()
            n212 = call-poly <vilib>:"WPI_RobotDriveArcadeDrive.vi"("error in (no error)"=w316, "Y axis value"=w310, "X axis value"=w311, "RobotDriveDevRef"=w317) -> ("error out"=w314:errorcluster, "Motor Values"=w318:dbl[], "RobotDriveDevRef"=w315:T1)  [unwired: 5 in]
            n213 = Equal?(x=2000, y=w308) -> (x = y?=w306:bool)
            n214 = global write "Robot Global Data.vi" "Motor Array"(w318) -> ()
            n215 = global write "Robot Global Data.vi" "RightMotors"(w310) -> ()
            n216 = Wait (ms)(milliseconds to wait=u32 1) -> ()  [unwired: 1 out]
          }
        }
        frame #2 {
          w321 = 0.0 ("LeftSpeed")
          n217 = call <vilib>:"WPI_RobotDriveMotors.vi"("error in (no error)"=w323, "RightSpeed"=w321, "LeftSpeed"=w321, "RobotDriveDevRef"=w324) -> ("Motor Values"=w320:dbl[])  [unwired: 5 in, 2 out]
          n218 = Wait (ms)(milliseconds to wait=u32 100) -> ()  [unwired: 1 out]
          n219 = global write "Robot Global Data.vi" "LeftMotors"(w321) -> ()
          n220 = global write "Robot Global Data.vi" "Motor Array"(w320) -> ()
          n221 = global write "Robot Global Data.vi" "RightMotors"(w321) -> ()
        }
      }
    }
    frame "Test Run 3" {
      n222 = flat-sequence {
        tunnel: [w333] -> w328
        tunnel: [w331] -> w327
        tunnel: w328 -> [w342]
        tunnel: w327 -> [w341]
        tunnel: [w340] -> w326
        tunnel: [w339] -> w325
        tunnel: w326 -> [w358]
        tunnel: w325 -> [w357]
        frame #0 {
          w330 = 0.0 ("TopLeftMotor")
          n223 = Wait (ms)(milliseconds to wait=u32 100) -> ()  [unwired: 1 out]
          n224 = global write "Robot Global Data.vi" "RightMotors"(w330) -> ()
          n225 = global write "Robot Global Data.vi" "LeftMotors"(w330) -> ()
          n226 = call <vilib>:"WPI_RobotDriveRefNum Registry Get.vi"("refnum name"="Motors") -> ("error out"=w333:errorcluster, "RobotDriveDevRef"=w332:T1)  [unwired: 9 in]
          n227 = call <vilib>:"WPI_RobotDriveMotors.vi"("RightSpeed"=w330, "LeftSpeed"=w330, "RobotDriveDevRef"=w332) -> ("Motor Values"=w329:dbl[], "RobotDriveDevRef"=w331:T1)  [unwired: 6 in, 1 out]
          n228 = global write "Robot Global Data.vi" "Motor Array"(w329) -> ()
          n229 = call <vilib>:"WPI_GyroRefNum Registry Get.vi"("refnum name"="My Gyro RefNum") -> ("error out"=w336:errorcluster, "GyroDevRef"=w337:T6)  [unwired: 9 in]
          n230 = call <vilib>:"WPI_GyroReset.vi"("error in"=w336, "GyroDevRef"=w337) -> ()  [unwired: 8 in, 2 out]
        }
        frame #1 {
          n231 = while {
            tunnel: w342 -> [w350]
            tunnel: w341 -> [w351]
            tunnel: [w349] -> w340
            tunnel: [w348] -> w339
            i -> [w346]
            stop <- w345 stop-if-true
            w343 = 0.5 ("LeftMotors")
            n232 = global read "Robot Global Data.vi" "RIGHT SPEED VARIABLE"() -> (w344:dbl)
            n233 = global write "Robot Global Data.vi" "LeftMotors"(w343) -> ()
            n234 = global write "Robot Global Data.vi" "RightMotors"(w344) -> ()
            n235 = call <vilib>:"WPI_RobotDriveTankDrive.vi"("error in (no error)"=w350, "Right axis value"=w344, "Left axis value"=w343, "RobotDriveDevRef"=w351) -> ("error out"=w348:errorcluster, "Motor Values"=w352:dbl[], "RobotDriveDevRef"=w349:T1)  [unwired: 5 in]
            n236 = global write "Robot Global Data.vi" "Motor Array"(w352) -> ()
            n237 = Equal?(x=2000, y=w346) -> (x = y?=w345:bool)
            n238 = Wait (ms)(milliseconds to wait=u32 1) -> ()  [unwired: 1 out]
          }
        }
        frame #2 {
          w355 = 0.0 ("LeftSpeed")
          n239 = call <vilib>:"WPI_RobotDriveMotors.vi"("error in (no error)"=w357, "RightSpeed"=w355, "LeftSpeed"=w355, "RobotDriveDevRef"=w358) -> ("Motor Values"=w354:dbl[])  [unwired: 5 in, 2 out]
          n240 = Wait (ms)(milliseconds to wait=u32 100) -> ()  [unwired: 1 out]
          n241 = global write "Robot Global Data.vi" "Motor Array"(w354) -> ()
          n242 = global write "Robot Global Data.vi" "LeftMotors"(w355) -> ()
          n243 = global write "Robot Global Data.vi" "RightMotors"(w355) -> ()
        }
      }
    }
    frame "Vision Test" {
      n244 = flat-sequence {
        tunnel: [w367] -> w362
        tunnel: [w365] -> w361
        tunnel: w362 -> [w376]
        tunnel: w361 -> [w375]
        tunnel: [w374] -> w360
        tunnel: [w373] -> w359
        tunnel: w360 -> [w391]
        tunnel: w359 -> [w390]
        frame #0 {
          w364 = 0.0 ("TopLeftMotor")
          n245 = Wait (ms)(milliseconds to wait=u32 100) -> ()  [unwired: 1 out]
          n246 = global write "Robot Global Data.vi" "RightMotors"(w364) -> ()
          n247 = global write "Robot Global Data.vi" "LeftMotors"(w364) -> ()
          n248 = call <vilib>:"WPI_RobotDriveRefNum Registry Get.vi"("refnum name"="Motors") -> ("error out"=w367:errorcluster, "RobotDriveDevRef"=w366:T1)  [unwired: 9 in]
          n249 = call <vilib>:"WPI_RobotDriveMotors.vi"("RightSpeed"=w364, "LeftSpeed"=w364, "RobotDriveDevRef"=w366) -> ("Motor Values"=w363:dbl[], "RobotDriveDevRef"=w365:T1)  [unwired: 6 in, 1 out]
          n250 = global write "Robot Global Data.vi" "Motor Array"(w363) -> ()
          n251 = call <vilib>:"WPI_GyroRefNum Registry Get.vi"("refnum name"="My Gyro RefNum") -> ("error out"=w370:errorcluster, "GyroDevRef"=w371:T6)  [unwired: 9 in]
          n252 = call <vilib>:"WPI_GyroReset.vi"("error in"=w370, "GyroDevRef"=w371) -> ()  [unwired: 8 in, 2 out]
        }
        frame #1 {
          n253 = while {
            tunnel: w376 -> [w379]
            tunnel: w375 -> [w380]
            tunnel: [w377] -> w374
            tunnel: [w378] -> w373
            stop <- FALSE stop-if-true
            # "into motor"
            n254 = global read "Robot Global Data.vi" "Vision Turn"() -> (w383:dbl)
            n255 = Negate(x=w383) -> (-x=w384:dbl)
            n256 = global write "Robot Global Data.vi" "LeftMotors"(w383) -> ()
            n257 = call <vilib>:"WPI_RobotDriveMotors.vi"("error in (no error)"=w379, "RightSpeed"=w384, "LeftSpeed"=w383, "RobotDriveDevRef"=w380) -> ("error out"=w378:errorcluster, "Motor Values"=w382:dbl[], "RobotDriveDevRef"=w377:T1)  [unwired: 5 out]
            n258 = global write "Robot Global Data.vi" "Vision needed"(TRUE ("Vision needed")) -> ()
            n259 = global write "Robot Global Data.vi" "Motor Array"(w382) -> ()
            n260 = global write "Robot Global Data.vi" "RightMotors"(w384) -> ()
            n261 = Wait (ms)(milliseconds to wait=u32 1) -> ()  [unwired: 1 out]
          }
        }
        frame #2 {
          w388 = 0.0 ("LeftSpeed")
          n262 = call <vilib>:"WPI_RobotDriveMotors.vi"("error in (no error)"=w390, "RightSpeed"=w388, "LeftSpeed"=w388, "RobotDriveDevRef"=w391) -> ("Motor Values"=w387:dbl[])  [unwired: 5 in, 2 out]
          n263 = Wait (ms)(milliseconds to wait=u32 100) -> ()  [unwired: 1 out]
          n264 = global write "Robot Global Data.vi" "LeftMotors"(w388) -> ()
          n265 = global write "Robot Global Data.vi" "Motor Array"(w387) -> ()
          n266 = global write "Robot Global Data.vi" "RightMotors"(w388) -> ()
        }
      }
    }
    frame "Vision Test 2" {
      n267 = flat-sequence {
        tunnel: [w400] -> w395
        tunnel: [w398] -> w394
        tunnel: w395 -> [w409]
        tunnel: w394 -> [w408]
        tunnel: [w407] -> w393
        tunnel: [w406] -> w392
        tunnel: w393 -> [w424]
        tunnel: w392 -> [w423]
        frame #0 {
          w397 = 0.0 ("TopLeftMotor")
          n268 = Wait (ms)(milliseconds to wait=u32 100) -> ()  [unwired: 1 out]
          n269 = global write "Robot Global Data.vi" "RightMotors"(w397) -> ()
          n270 = global write "Robot Global Data.vi" "LeftMotors"(w397) -> ()
          n271 = call <vilib>:"WPI_RobotDriveRefNum Registry Get.vi"("refnum name"="Motors") -> ("error out"=w400:errorcluster, "RobotDriveDevRef"=w399:T1)  [unwired: 9 in]
          n272 = call <vilib>:"WPI_RobotDriveMotors.vi"("RightSpeed"=w397, "LeftSpeed"=w397, "RobotDriveDevRef"=w399) -> ("Motor Values"=w396:dbl[], "RobotDriveDevRef"=w398:T1)  [unwired: 6 in, 1 out]
          n273 = global write "Robot Global Data.vi" "Motor Array"(w396) -> ()
          n274 = call <vilib>:"WPI_GyroRefNum Registry Get.vi"("refnum name"="My Gyro RefNum") -> ("error out"=w403:errorcluster, "GyroDevRef"=w404:T6)  [unwired: 9 in]
          n275 = call <vilib>:"WPI_GyroReset.vi"("error in"=w403, "GyroDevRef"=w404) -> ()  [unwired: 8 in, 2 out]
        }
        frame #1 {
          n276 = while {
            tunnel: w409 -> [w414]
            tunnel: w408 -> [w415]
            tunnel: [w412] -> w407
            tunnel: [w413] -> w406
            stop <- FALSE stop-if-true
            w410 = 0.0 ("Y axis value")
            # "into arcade"
            n277 = global read "Robot Global Data.vi" "Vision Turn"() -> (w411:dbl)
            n278 = global write "Robot Global Data.vi" "RightMotors"(w410) -> ()
            n279 = global write "Robot Global Data.vi" "LeftMotors"(w411) -> ()
            n280 = call-poly <vilib>:"WPI_RobotDriveArcadeDrive.vi"("error in (no error)"=w414, "Y axis value"=w410, "X axis value"=w411, "RobotDriveDevRef"=w415) -> ("error out"=w413:errorcluster, "Motor Values"=w417:dbl[], "RobotDriveDevRef"=w412:T1)  [unwired: 5 in]
            n281 = global write "Robot Global Data.vi" "Vision needed"(TRUE ("Vision needed")) -> ()
            n282 = global write "Robot Global Data.vi" "Motor Array"(w417) -> ()
            n283 = Wait (ms)(milliseconds to wait=u32 1) -> ()  [unwired: 1 out]
          }
        }
        frame #2 {
          w421 = 0.0 ("LeftSpeed")
          n284 = call <vilib>:"WPI_RobotDriveMotors.vi"("error in (no error)"=w423, "RightSpeed"=w421, "LeftSpeed"=w421, "RobotDriveDevRef"=w424) -> ("Motor Values"=w420:dbl[])  [unwired: 5 in, 2 out]
          n285 = Wait (ms)(milliseconds to wait=u32 100) -> ()  [unwired: 1 out]
          n286 = global write "Robot Global Data.vi" "LeftMotors"(w421) -> ()
          n287 = global write "Robot Global Data.vi" "Motor Array"(w420) -> ()
          n288 = global write "Robot Global Data.vi" "RightMotors"(w421) -> ()
        }
      }
    }
    frame "Vision Test 3" {
      n289 = flat-sequence {
        tunnel: [w433] -> w428
        tunnel: [w431] -> w427
        tunnel: w428 -> [w442]
        tunnel: w427 -> [w441]
        tunnel: [w440] -> w426
        tunnel: [w439] -> w425
        tunnel: w426 -> [w457]
        tunnel: w425 -> [w456]
        frame #0 {
          w430 = 0.0 ("TopLeftMotor")
          n290 = Wait (ms)(milliseconds to wait=u32 100) -> ()  [unwired: 1 out]
          n291 = global write "Robot Global Data.vi" "RightMotors"(w430) -> ()
          n292 = global write "Robot Global Data.vi" "LeftMotors"(w430) -> ()
          n293 = call <vilib>:"WPI_RobotDriveRefNum Registry Get.vi"("refnum name"="Motors") -> ("error out"=w433:errorcluster, "RobotDriveDevRef"=w432:T1)  [unwired: 9 in]
          n294 = call <vilib>:"WPI_RobotDriveMotors.vi"("RightSpeed"=w430, "LeftSpeed"=w430, "RobotDriveDevRef"=w432) -> ("Motor Values"=w429:dbl[], "RobotDriveDevRef"=w431:T1)  [unwired: 6 in, 1 out]
          n295 = global write "Robot Global Data.vi" "Motor Array"(w429) -> ()
          n296 = call <vilib>:"WPI_GyroRefNum Registry Get.vi"("refnum name"="My Gyro RefNum") -> ("error out"=w436:errorcluster, "GyroDevRef"=w437:T6)  [unwired: 9 in]
          n297 = call <vilib>:"WPI_GyroReset.vi"("error in"=w436, "GyroDevRef"=w437) -> ()  [unwired: 8 in, 2 out]
        }
        frame #1 {
          n298 = while {
            tunnel: w442 -> [w445]
            tunnel: w441 -> [w446]
            tunnel: [w443] -> w440
            tunnel: [w444] -> w439
            stop <- FALSE stop-if-true
            # "Tank drive"
            n299 = global read "Robot Global Data.vi" "Vision Turn"() -> (w449:dbl)
            n300 = Negate(x=w449) -> (-x=w450:dbl)
            n301 = global write "Robot Global Data.vi" "LeftMotors"(w449) -> ()
            n302 = call <vilib>:"WPI_RobotDriveTankDrive.vi"("error in (no error)"=w445, "Right axis value"=w450, "Left axis value"=w449, "RobotDriveDevRef"=w446) -> ("error out"=w444:errorcluster, "Motor Values"=w448:dbl[], "RobotDriveDevRef"=w443:T1)  [unwired: 5 in]
            n303 = global write "Robot Global Data.vi" "Vision needed"(TRUE ("Vision needed")) -> ()
            n304 = global write "Robot Global Data.vi" "Motor Array"(w448) -> ()
            n305 = global write "Robot Global Data.vi" "RightMotors"(w450) -> ()
            n306 = Wait (ms)(milliseconds to wait=u32 1) -> ()  [unwired: 1 out]
          }
        }
        frame #2 {
          w454 = 0.0 ("LeftSpeed")
          n307 = call <vilib>:"WPI_RobotDriveMotors.vi"("error in (no error)"=w456, "RightSpeed"=w454, "LeftSpeed"=w454, "RobotDriveDevRef"=w457) -> ("Motor Values"=w453:dbl[])  [unwired: 5 in, 2 out]
          n308 = Wait (ms)(milliseconds to wait=u32 100) -> ()  [unwired: 1 out]
          n309 = global write "Robot Global Data.vi" "LeftMotors"(w454) -> ()
          n310 = global write "Robot Global Data.vi" "Motor Array"(w453) -> ()
          n311 = global write "Robot Global Data.vi" "RightMotors"(w454) -> ()
        }
      }
    }
    frame "Vision Test 4" {
      n312 = flat-sequence {
        tunnel: [w466] -> w461
        tunnel: [w464] -> w460
        tunnel: w461 -> [w474]
        tunnel: w460 -> [w475]
        tunnel: [w473] -> w459
        tunnel: [w472] -> w458
        tunnel: w459 -> [w493]
        tunnel: w458 -> [w492]
        frame #0 {
          w463 = 0.0 ("TopLeftMotor")
          n313 = Wait (ms)(milliseconds to wait=u32 100) -> ()  [unwired: 1 out]
          n314 = global write "Robot Global Data.vi" "RightMotors"(w463) -> ()
          n315 = global write "Robot Global Data.vi" "LeftMotors"(w463) -> ()
          n316 = call <vilib>:"WPI_RobotDriveRefNum Registry Get.vi"("refnum name"="Motors") -> ("error out"=w466:errorcluster, "RobotDriveDevRef"=w465:T1)  [unwired: 9 in]
          n317 = call <vilib>:"WPI_RobotDriveMotors.vi"("RightSpeed"=w463, "LeftSpeed"=w463, "RobotDriveDevRef"=w465) -> ("Motor Values"=w462:dbl[], "RobotDriveDevRef"=w464:T1)  [unwired: 6 in, 1 out]
          n318 = global write "Robot Global Data.vi" "Motor Array"(w462) -> ()
          n319 = call <vilib>:"WPI_GyroRefNum Registry Get.vi"("refnum name"="My Gyro RefNum") -> ("error out"=w469:errorcluster, "GyroDevRef"=w470:T6)  [unwired: 9 in]
          n320 = call <vilib>:"WPI_GyroReset.vi"("error in"=w469, "GyroDevRef"=w470) -> ()  [unwired: 8 in, 2 out]
        }
        frame #1 {
          n321 = while {
            tunnel: w475 -> [w481]
            tunnel: w474 -> [w482]
            tunnel: [w478] -> w473
            tunnel: [w477] -> w472
            stop <- FALSE stop-if-true
            n322 = global read "Robot Global Data.vi" "GyroAngle"() -> (w483:dbl)
            n323 = global write "Robot Global Data.vi" "Gyro Rest?"(FALSE ("Gyro Rest?")) -> ()
            n324 = global read "Robot Global Data.vi" "X?"() -> (w484:dbl)
            n325 = call "vision sub.vi"("Gyro Angle"=w483, "X? Input"=w484) -> ("Right Motors"=w487:dbl, "Left Motors"=w488:dbl, "Nothing In Sight"=w486:bool)  [unwired: 7 in]
            n326 = global write "Robot Global Data.vi" "Vision Nothing In Sight"(w486) -> ()
            n327 = call <vilib>:"WPI_RobotDriveMotors.vi"("error in (no error)"=w482, "RightSpeed"=w487, "LeftSpeed"=w488, "RobotDriveDevRef"=w481) -> ("error out"=w477:errorcluster, "Motor Values"=w485:dbl[], "RobotDriveDevRef"=w478:T1)  [unwired: 5 out]
            n328 = global write "Robot Global Data.vi" "RightMotors"(w487) -> ()
            n329 = global write "Robot Global Data.vi" "LeftMotors"(w488) -> ()
            n330 = global write "Robot Global Data.vi" "Motor Array"(w485) -> ()
          }
          n331 = global write "Robot Global Data.vi" "Gyro Rest?"(TRUE ("Gyro Rest?")) -> ()
        }
        frame #2 {
          w490 = 0.0 ("LeftSpeed")
          n332 = call <vilib>:"WPI_RobotDriveMotors.vi"("error in (no error)"=w492, "RightSpeed"=w490, "LeftSpeed"=w490, "RobotDriveDevRef"=w493) -> ("Motor Values"=w489:dbl[])  [unwired: 5 in, 2 out]
          n333 = Wait (ms)(milliseconds to wait=u32 100) -> ()  [unwired: 1 out]
          n334 = global write "Robot Global Data.vi" "LeftMotors"(w490) -> ()
          n335 = global write "Robot Global Data.vi" "Motor Array"(w489) -> ()
          n336 = global write "Robot Global Data.vi" "RightMotors"(w490) -> ()
        }
      }
    }
    frame "VisionGyro Forward" {
      n337 = flat-sequence {
        tunnel: [w504] -> w499
        tunnel: [w502] -> w498
        tunnel: w499 -> [w513]
        tunnel: w498 -> [w512]
        tunnel: [w511] -> w497
        tunnel: [w510] -> w496
        tunnel: w497 -> [w545]
        tunnel: w496 -> [w544]
        tunnel: [w540] -> w495
        tunnel: [w539] -> w494
        tunnel: w495 -> [w548]
        tunnel: w494 -> [w547]
        frame #0 {
          w501 = 0.0 ("TopLeftMotor")
          n338 = Wait (ms)(milliseconds to wait=u32 100) -> ()  [unwired: 1 out]
          n339 = global write "Robot Global Data.vi" "RightMotors"(w501) -> ()
          n340 = global write "Robot Global Data.vi" "LeftMotors"(w501) -> ()
          n341 = call <vilib>:"WPI_RobotDriveRefNum Registry Get.vi"("refnum name"="Motors") -> ("error out"=w504:errorcluster, "RobotDriveDevRef"=w503:T1)  [unwired: 9 in]
          n342 = call <vilib>:"WPI_RobotDriveMotors.vi"("RightSpeed"=w501, "LeftSpeed"=w501, "RobotDriveDevRef"=w503) -> ("Motor Values"=w500:dbl[], "RobotDriveDevRef"=w502:T1)  [unwired: 6 in, 1 out]
          n343 = global write "Robot Global Data.vi" "Motor Array"(w500) -> ()
          n344 = call <vilib>:"WPI_GyroRefNum Registry Get.vi"("refnum name"="My Gyro RefNum") -> ("error out"=w507:errorcluster, "GyroDevRef"=w508:T6)  [unwired: 9 in]
          n345 = call <vilib>:"WPI_GyroReset.vi"("error in"=w507, "GyroDevRef"=w508) -> ()  [unwired: 8 in, 2 out]
        }
        frame #1 {
          n346 = while {
            tunnel: w513 -> [w533]
            tunnel: w512 -> [w534]
            tunnel: [w532] -> w511
            tunnel: [w531] -> w510
            i -> [w517]
            stop <- w516 stop-if-true
            n347 = global read "Robot Global Data.vi" "GyroAngle"() -> (w519:dbl)
            n348 = global read "Robot Global Data.vi" "Autonomos Gyro forward SPEED VARIABLE"() -> (w515:dbl)
            n349 = expression code="(x/180.0)*pi" "degrees to radians"(w519) -> (w518:dbl)
            n350 = Negate(x=w518) -> (-x=w524:dbl)
            n351 = Sine(x=w524) -> (sin(x)=w526:dbl)
            n352 = Sine(x=w518) -> (sin(x)=w528:dbl)
            n353 = Increment(x=w526) -> (x+1=w525:dbl)
            n354 = Increment(x=w528) -> (x+1=w527:dbl)
            n355 = Max & Min(x=w525, y=1.0) -> (min(x,y)=w522:dbl)  [unwired: 1 out]
            n356 = Max & Min(x=1.0, y=w527) -> (min(x,y)=w523:dbl)  [unwired: 1 out]
            n357 = global read "Robot Global Data.vi" "Autonoums Delay"() -> (w514:dbl)
            n358 = Multiply(x=w515, y=w522) -> (x*y=w521:dbl)
            n359 = Multiply(x=w515, y=w523) -> (x*y=w520:dbl)
            n360 = Negate(x=w521) -> (-x=w535:dbl)
            n361 = Negate(x=w520) -> (-x=w536:dbl)
            n362 = Equal?(x=w517, y=w514) -> (x = y?=w516:bool)
            n363 = call <vilib>:"WPI_RobotDriveMotors.vi"("error in (no error)"=w533, "RightSpeed"=w536, "LeftSpeed"=w535, "RobotDriveDevRef"=w534) -> ("error out"=w531:errorcluster, "Motor Values"=w537:dbl[], "RobotDriveDevRef"=w532:T1)  [unwired: 5 in]
            n364 = Wait (ms)(milliseconds to wait=u32 1) -> ()  [unwired: 1 out]
            n365 = global write "Robot Global Data.vi" "LeftMotors"(w535) -> ()
            n366 = global write "Robot Global Data.vi" "Motor Array"(w537) -> ()
            n367 = global write "Robot Global Data.vi" "RightMotors"(w536) -> ()
          }
        }
        frame #2 {
          w542 = 0.0 ("LeftSpeed")
          n368 = call <vilib>:"WPI_RobotDriveMotors.vi"("error in (no error)"=w544, "RightSpeed"=w542, "LeftSpeed"=w542, "RobotDriveDevRef"=w545) -> ("error out"=w539:errorcluster, "Motor Values"=w541:dbl[], "RobotDriveDevRef"=w540:T1)  [unwired: 5 in]
          n369 = Wait (ms)(milliseconds to wait=u32 100) -> ()  [unwired: 1 out]
          n370 = global write "Robot Global Data.vi" "LeftMotors"(w542) -> ()
          n371 = global write "Robot Global Data.vi" "Motor Array"(w541) -> ()
          n372 = global write "Robot Global Data.vi" "RightMotors"(w542) -> ()
        }
        frame #3 {
          n373 = while {
            tunnel: w548 -> [w551]
            tunnel: w547 -> [w552]
            stop <- FALSE stop-if-true
            n374 = global read "Robot Global Data.vi" "GyroAngle"() -> (w553:dbl)
            n375 = global write "Robot Global Data.vi" "Gyro Rest?"(FALSE ("Gyro Rest?")) -> ()
            n376 = global read "Robot Global Data.vi" "X?"() -> (w554:dbl)
            n377 = call "vision sub.vi"("Gyro Angle"=w553, "X? Input"=w554) -> ("Right Motors"=w557:dbl, "Left Motors"=w558:dbl, "Nothing In Sight"=w556:bool)  [unwired: 7 in]
            n378 = global write "Robot Global Data.vi" "Vision Nothing In Sight"(w556) -> ()
            n379 = call <vilib>:"WPI_RobotDriveMotors.vi"("error in (no error)"=w552, "RightSpeed"=w557, "LeftSpeed"=w558, "RobotDriveDevRef"=w551) -> ("Motor Values"=w555:dbl[])  [unwired: 7 out]
            n380 = global write "Robot Global Data.vi" "RightMotors"(w557) -> ()
            n381 = global write "Robot Global Data.vi" "LeftMotors"(w558) -> ()
            n382 = global write "Robot Global Data.vi" "Motor Array"(w555) -> ()
          }
          n383 = global write "Robot Global Data.vi" "Gyro Rest?"(TRUE ("Gyro Rest?")) -> ()
        }
      }
    }
    frame "VisionGyro Both Sides" {
      n384 = flat-sequence {
        tunnel: [w569] -> w564
        tunnel: [w567] -> w563
        tunnel: w564 -> [w578]
        tunnel: w563 -> [w577]
        tunnel: [w576] -> w562
        tunnel: [w575] -> w561
        tunnel: w562 -> [w612]
        tunnel: w561 -> [w611]
        tunnel: [w607] -> w560
        tunnel: [w606] -> w559
        tunnel: w560 -> [w615]
        tunnel: w559 -> [w614]
        frame #0 {
          w566 = 0.0 ("TopLeftMotor")
          n385 = Wait (ms)(milliseconds to wait=u32 100) -> ()  [unwired: 1 out]
          n386 = global write "Robot Global Data.vi" "RightMotors"(w566) -> ()
          n387 = global write "Robot Global Data.vi" "LeftMotors"(w566) -> ()
          n388 = call <vilib>:"WPI_RobotDriveRefNum Registry Get.vi"("refnum name"="Motors") -> ("error out"=w569:errorcluster, "RobotDriveDevRef"=w568:T1)  [unwired: 9 in]
          n389 = call <vilib>:"WPI_RobotDriveMotors.vi"("RightSpeed"=w566, "LeftSpeed"=w566, "RobotDriveDevRef"=w568) -> ("Motor Values"=w565:dbl[], "RobotDriveDevRef"=w567:T1)  [unwired: 6 in, 1 out]
          n390 = global write "Robot Global Data.vi" "Motor Array"(w565) -> ()
          n391 = call <vilib>:"WPI_GyroRefNum Registry Get.vi"("refnum name"="My Gyro RefNum") -> ("error out"=w572:errorcluster, "GyroDevRef"=w573:T6)  [unwired: 9 in]
          n392 = call <vilib>:"WPI_GyroReset.vi"("error in"=w572, "GyroDevRef"=w573) -> ()  [unwired: 8 in, 2 out]
        }
        frame #1 {
          n393 = while {
            tunnel: w578 -> [w600]
            tunnel: w577 -> [w601]
            tunnel: [w599] -> w576
            tunnel: [w598] -> w575
            i -> [w584]
            stop <- w583 stop-if-true
            n394 = global read "Robot Global Data.vi" "GyroAngle"() -> (w586:dbl)
            n395 = global read "Robot Global Data.vi" "Autonomos Gyro forward SPEED VARIABLE"() -> (w582:dbl)
            n396 = expression code="(x/180.0)*pi" "degrees to radians"(w586) -> (w585:dbl)
            n397 = Negate(x=w585) -> (-x=w591:dbl)
            n398 = Sine(x=w591) -> (sin(x)=w593:dbl)
            n399 = Sine(x=w585) -> (sin(x)=w595:dbl)
            n400 = Increment(x=w593) -> (x+1=w592:dbl)
            n401 = Increment(x=w595) -> (x+1=w594:dbl)
            n402 = Max & Min(x=w592, y=1.0) -> (min(x,y)=w589:dbl)  [unwired: 1 out]
            n403 = Max & Min(x=1.0, y=w594) -> (min(x,y)=w590:dbl)  [unwired: 1 out]
            n404 = global read "Robot Global Data.vi" "Autonoums Delay"() -> (w581:dbl)
            n405 = Multiply(x=w582, y=w589) -> (x*y=w588:dbl)
            n406 = Multiply(x=w582, y=w590) -> (x*y=w587:dbl)
            n407 = Add(x=w581, y=1000.0) -> (x+y=w580:dbl)
            n408 = Negate(x=w588) -> (-x=w602:dbl)
            n409 = Negate(x=w587) -> (-x=w603:dbl)
            n410 = Equal?(x=w584, y=w580) -> (x = y?=w583:bool)
            n411 = call <vilib>:"WPI_RobotDriveMotors.vi"("error in (no error)"=w600, "RightSpeed"=w603, "LeftSpeed"=w602, "RobotDriveDevRef"=w601) -> ("error out"=w598:errorcluster, "Motor Values"=w604:dbl[], "RobotDriveDevRef"=w599:T1)  [unwired: 5 in]
            n412 = Wait (ms)(milliseconds to wait=u32 1) -> ()  [unwired: 1 out]
            n413 = global write "Robot Global Data.vi" "LeftMotors"(w602) -> ()
            n414 = global write "Robot Global Data.vi" "Motor Array"(w604) -> ()
            n415 = global write "Robot Global Data.vi" "RightMotors"(w603) -> ()
          }
        }
        frame #2 {
          w609 = 0.0 ("LeftSpeed")
          n416 = call <vilib>:"WPI_RobotDriveMotors.vi"("error in (no error)"=w611, "RightSpeed"=w609, "LeftSpeed"=w609, "RobotDriveDevRef"=w612) -> ("error out"=w606:errorcluster, "Motor Values"=w608:dbl[], "RobotDriveDevRef"=w607:T1)  [unwired: 5 in]
          n417 = Wait (ms)(milliseconds to wait=u32 100) -> ()  [unwired: 1 out]
          n418 = global write "Robot Global Data.vi" "LeftMotors"(w609) -> ()
          n419 = global write "Robot Global Data.vi" "Motor Array"(w608) -> ()
          n420 = global write "Robot Global Data.vi" "RightMotors"(w609) -> ()
        }
        frame #3 {
          n421 = while {
            tunnel: w615 -> [w618]
            tunnel: w614 -> [w619]
            stop <- FALSE stop-if-true
            n422 = global read "Robot Global Data.vi" "GyroAngle"() -> (w620:dbl)
            n423 = global write "Robot Global Data.vi" "Gyro Rest?"(FALSE ("Gyro Rest?")) -> ()
            n424 = global read "Robot Global Data.vi" "X?"() -> (w621:dbl)
            n425 = call "vision sub.vi"("Gyro Angle"=w620, "X? Input"=w621) -> ("Right Motors"=w624:dbl, "Left Motors"=w625:dbl, "Nothing In Sight"=w623:bool)  [unwired: 7 in]
            n426 = global write "Robot Global Data.vi" "Vision Nothing In Sight"(w623) -> ()
            n427 = call <vilib>:"WPI_RobotDriveMotors.vi"("error in (no error)"=w619, "RightSpeed"=w624, "LeftSpeed"=w625, "RobotDriveDevRef"=w618) -> ("Motor Values"=w622:dbl[])  [unwired: 7 out]
            n428 = global write "Robot Global Data.vi" "RightMotors"(w624) -> ()
            n429 = global write "Robot Global Data.vi" "LeftMotors"(w625) -> ()
            n430 = global write "Robot Global Data.vi" "Motor Array"(w622) -> ()
          }
          n431 = global write "Robot Global Data.vi" "Gyro Rest?"(TRUE ("Gyro Rest?")) -> ()
        }
      }
    }
    frame "VisionAngle Turn Right" {
      n432 = flat-sequence {
        tunnel: [w638] -> w633
        tunnel: [w636] -> w632
        tunnel: w633 -> [w647]
        tunnel: w632 -> [w646]
        tunnel: [w645] -> w631
        tunnel: [w644] -> w630
        tunnel: w631 -> [w681]
        tunnel: w630 -> [w680]
        tunnel: [w676] -> w629
        tunnel: [w675] -> w628
        tunnel: w629 -> [w685]
        tunnel: w628 -> [w684]
        tunnel: [w683] -> w627
        tunnel: [w682] -> w626
        tunnel: w627 -> [w699]
        tunnel: w626 -> [w698]
        frame #0 {
          w635 = 0.0 ("TopLeftMotor")
          n433 = Wait (ms)(milliseconds to wait=u32 100) -> ()  [unwired: 1 out]
          n434 = global write "Robot Global Data.vi" "RightMotors"(w635) -> ()
          n435 = global write "Robot Global Data.vi" "LeftMotors"(w635) -> ()
          n436 = call <vilib>:"WPI_RobotDriveRefNum Registry Get.vi"("refnum name"="Motors") -> ("error out"=w638:errorcluster, "RobotDriveDevRef"=w637:T1)  [unwired: 9 in]
          n437 = call <vilib>:"WPI_RobotDriveMotors.vi"("RightSpeed"=w635, "LeftSpeed"=w635, "RobotDriveDevRef"=w637) -> ("Motor Values"=w634:dbl[], "RobotDriveDevRef"=w636:T1)  [unwired: 6 in, 1 out]
          n438 = global write "Robot Global Data.vi" "Motor Array"(w634) -> ()
          n439 = call <vilib>:"WPI_GyroRefNum Registry Get.vi"("refnum name"="My Gyro RefNum") -> ("error out"=w641:errorcluster, "GyroDevRef"=w642:T6)  [unwired: 9 in]
          n440 = call <vilib>:"WPI_GyroReset.vi"("error in"=w641, "GyroDevRef"=w642) -> ()  [unwired: 8 in, 2 out]
        }
        frame #1 {
          n441 = while {
            tunnel: w647 -> [w669]
            tunnel: w646 -> [w670]
            tunnel: [w668] -> w645
            tunnel: [w667] -> w644
            i -> [w653]
            stop <- w652 stop-if-true
            n442 = global read "Robot Global Data.vi" "GyroAngle"() -> (w655:dbl)
            n443 = global read "Robot Global Data.vi" "Autonomos Gyro forward SPEED VARIABLE"() -> (w651:dbl)
            n444 = expression code="(x/180.0)*pi" "degrees to radians"(w655) -> (w654:dbl)
            n445 = Negate(x=w654) -> (-x=w660:dbl)
            n446 = Sine(x=w660) -> (sin(x)=w662:dbl)
            n447 = Sine(x=w654) -> (sin(x)=w664:dbl)
            n448 = Increment(x=w662) -> (x+1=w661:dbl)
            n449 = Increment(x=w664) -> (x+1=w663:dbl)
            n450 = Max & Min(x=w661, y=1.0) -> (min(x,y)=w658:dbl)  [unwired: 1 out]
            n451 = Max & Min(x=1.0, y=w663) -> (min(x,y)=w659:dbl)  [unwired: 1 out]
            n452 = global read "Robot Global Data.vi" "Autonoums Delay"() -> (w650:dbl)
            n453 = Multiply(x=w651, y=w658) -> (x*y=w657:dbl)
            n454 = Multiply(x=w651, y=w659) -> (x*y=w656:dbl)
            n455 = Negate(x=w657) -> (-x=w671:dbl)
            n456 = Negate(x=w656) -> (-x=w672:dbl)
            n457 = Add(x=w650, y=1000.0) -> (x+y=w649:dbl)
            n458 = Equal?(x=w653, y=w649) -> (x = y?=w652:bool)
            n459 = call <vilib>:"WPI_RobotDriveMotors.vi"("error in (no error)"=w669, "RightSpeed"=w672, "LeftSpeed"=w671, "RobotDriveDevRef"=w670) -> ("error out"=w667:errorcluster, "Motor Values"=w673:dbl[], "RobotDriveDevRef"=w668:T1)  [unwired: 5 in]
            n460 = Wait (ms)(milliseconds to wait=u32 1) -> ()  [unwired: 1 out]
            n461 = global write "Robot Global Data.vi" "LeftMotors"(w671) -> ()
            n462 = global write "Robot Global Data.vi" "Motor Array"(w673) -> ()
            n463 = global write "Robot Global Data.vi" "RightMotors"(w672) -> ()
          }
        }
        frame #2 {
          w678 = 0.0 ("LeftSpeed")
          n464 = call <vilib>:"WPI_RobotDriveMotors.vi"("error in (no error)"=w680, "RightSpeed"=w678, "LeftSpeed"=w678, "RobotDriveDevRef"=w681) -> ("error out"=w675:errorcluster, "Motor Values"=w677:dbl[], "RobotDriveDevRef"=w676:T1)  [unwired: 5 in]
          n465 = Wait (ms)(milliseconds to wait=u32 100) -> ()  [unwired: 1 out]
          n466 = global write "Robot Global Data.vi" "LeftMotors"(w678) -> ()
          n467 = global write "Robot Global Data.vi" "Motor Array"(w677) -> ()
          n468 = global write "Robot Global Data.vi" "RightMotors"(w678) -> ()
        }
        frame #3 {
          n469 = global write "Robot Global Data.vi" "Gyro Rest?"(TRUE ("Gyro Rest?")) -> ()
          n470 = while {
            tunnel: w685 -> [w689]
            tunnel: w684 -> [w690]
            tunnel: [w688] -> w683
            tunnel: [w687] -> w682
            stop <- w694 stop-if-true
            n471 = global write "Robot Global Data.vi" "Gyro Rest?"(FALSE ("Gyro Rest?")) -> ()
            n472 = global read "Robot Global Data.vi" "LEFT SPEED VARIABLE"() -> (w696:dbl)
            n473 = global read "Robot Global Data.vi" "GyroAngle"() -> (w692:dbl)
            n474 = call <vilib>:"WPI_RobotDriveMotors.vi"("error in (no error)"=w690, "RightSpeed"=w696, "LeftSpeed"=0.0, "RobotDriveDevRef"=w689) -> ("error out"=w687:errorcluster, "RobotDriveDevRef"=w688:T1)  [unwired: 5 in, 1 out]
            n475 = Equal?(x=w692, y=40.0) -> (x = y?=w694:bool)
          }
        }
        frame #4 {
          n476 = while {
            tunnel: w699 -> [w702]
            tunnel: w698 -> [w701]
            stop <- FALSE stop-if-true
            n477 = global read "Robot Global Data.vi" "GyroAngle"() -> (w704:dbl)
            n478 = global write "Robot Global Data.vi" "Gyro Rest?"(FALSE ("Gyro Rest?")) -> ()
            n479 = global read "Robot Global Data.vi" "X?"() -> (w705:dbl)
            n480 = call "vision sub.vi"("Gyro Angle"=w704, "X? Input"=w705) -> ("Right Motors"=w708:dbl, "Left Motors"=w709:dbl, "Nothing In Sight"=w707:bool)  [unwired: 7 in]
            n481 = global write "Robot Global Data.vi" "Vision Nothing In Sight"(w707) -> ()
            n482 = call <vilib>:"WPI_RobotDriveMotors.vi"("error in (no error)"=w701, "RightSpeed"=w708, "LeftSpeed"=w709, "RobotDriveDevRef"=w702) -> ("Motor Values"=w706:dbl[])  [unwired: 7 out]
            n483 = global write "Robot Global Data.vi" "RightMotors"(w708) -> ()
            n484 = global write "Robot Global Data.vi" "LeftMotors"(w709) -> ()
            n485 = global write "Robot Global Data.vi" "Motor Array"(w706) -> ()
          }
          n486 = global write "Robot Global Data.vi" "Gyro Rest?"(TRUE ("Gyro Rest?")) -> ()
        }
      }
    }
    frame "VisionAngle Turn Left" {
      n487 = flat-sequence {
        tunnel: [w722] -> w717
        tunnel: [w720] -> w716
        tunnel: w717 -> [w731]
        tunnel: w716 -> [w730]
        tunnel: [w729] -> w715
        tunnel: [w728] -> w714
        tunnel: w715 -> [w765]
        tunnel: w714 -> [w764]
        tunnel: [w760] -> w713
        tunnel: [w759] -> w712
        tunnel: w713 -> [w769]
        tunnel: w712 -> [w768]
        tunnel: [w767] -> w711
        tunnel: [w766] -> w710
        tunnel: w711 -> [w783]
        tunnel: w710 -> [w782]
        frame #0 {
          w719 = 0.0 ("TopLeftMotor")
          n488 = Wait (ms)(milliseconds to wait=u32 100) -> ()  [unwired: 1 out]
          n489 = global write "Robot Global Data.vi" "RightMotors"(w719) -> ()
          n490 = global write "Robot Global Data.vi" "LeftMotors"(w719) -> ()
          n491 = call <vilib>:"WPI_RobotDriveRefNum Registry Get.vi"("refnum name"="Motors") -> ("error out"=w722:errorcluster, "RobotDriveDevRef"=w721:T1)  [unwired: 9 in]
          n492 = call <vilib>:"WPI_RobotDriveMotors.vi"("RightSpeed"=w719, "LeftSpeed"=w719, "RobotDriveDevRef"=w721) -> ("Motor Values"=w718:dbl[], "RobotDriveDevRef"=w720:T1)  [unwired: 6 in, 1 out]
          n493 = global write "Robot Global Data.vi" "Motor Array"(w718) -> ()
          n494 = call <vilib>:"WPI_GyroRefNum Registry Get.vi"("refnum name"="My Gyro RefNum") -> ("error out"=w725:errorcluster, "GyroDevRef"=w726:T6)  [unwired: 9 in]
          n495 = call <vilib>:"WPI_GyroReset.vi"("error in"=w725, "GyroDevRef"=w726) -> ()  [unwired: 8 in, 2 out]
        }
        frame #1 {
          n496 = while {
            tunnel: w731 -> [w753]
            tunnel: w730 -> [w754]
            tunnel: [w752] -> w729
            tunnel: [w751] -> w728
            i -> [w737]
            stop <- w736 stop-if-true
            n497 = global read "Robot Global Data.vi" "GyroAngle"() -> (w739:dbl)
            n498 = global read "Robot Global Data.vi" "Autonomos Gyro forward SPEED VARIABLE"() -> (w735:dbl)
            n499 = expression code="(x/180.0)*pi" "degrees to radians"(w739) -> (w738:dbl)
            n500 = Negate(x=w738) -> (-x=w744:dbl)
            n501 = Sine(x=w744) -> (sin(x)=w746:dbl)
            n502 = Sine(x=w738) -> (sin(x)=w748:dbl)
            n503 = Increment(x=w746) -> (x+1=w745:dbl)
            n504 = Increment(x=w748) -> (x+1=w747:dbl)
            n505 = Max & Min(x=w745, y=1.0) -> (min(x,y)=w742:dbl)  [unwired: 1 out]
            n506 = Max & Min(x=1.0, y=w747) -> (min(x,y)=w743:dbl)  [unwired: 1 out]
            n507 = global read "Robot Global Data.vi" "Autonoums Delay"() -> (w734:dbl)
            n508 = Multiply(x=w735, y=w742) -> (x*y=w741:dbl)
            n509 = Multiply(x=w735, y=w743) -> (x*y=w740:dbl)
            n510 = Negate(x=w741) -> (-x=w755:dbl)
            n511 = Negate(x=w740) -> (-x=w756:dbl)
            n512 = Add(x=w734, y=1000.0) -> (x+y=w733:dbl)
            n513 = Equal?(x=w737, y=w733) -> (x = y?=w736:bool)
            n514 = call <vilib>:"WPI_RobotDriveMotors.vi"("error in (no error)"=w753, "RightSpeed"=w756, "LeftSpeed"=w755, "RobotDriveDevRef"=w754) -> ("error out"=w751:errorcluster, "Motor Values"=w757:dbl[], "RobotDriveDevRef"=w752:T1)  [unwired: 5 in]
            n515 = Wait (ms)(milliseconds to wait=u32 1) -> ()  [unwired: 1 out]
            n516 = global write "Robot Global Data.vi" "LeftMotors"(w755) -> ()
            n517 = global write "Robot Global Data.vi" "Motor Array"(w757) -> ()
            n518 = global write "Robot Global Data.vi" "RightMotors"(w756) -> ()
          }
        }
        frame #2 {
          w762 = 0.0 ("LeftSpeed")
          n519 = call <vilib>:"WPI_RobotDriveMotors.vi"("error in (no error)"=w764, "RightSpeed"=w762, "LeftSpeed"=w762, "RobotDriveDevRef"=w765) -> ("error out"=w759:errorcluster, "Motor Values"=w761:dbl[], "RobotDriveDevRef"=w760:T1)  [unwired: 5 in]
          n520 = Wait (ms)(milliseconds to wait=u32 100) -> ()  [unwired: 1 out]
          n521 = global write "Robot Global Data.vi" "LeftMotors"(w762) -> ()
          n522 = global write "Robot Global Data.vi" "Motor Array"(w761) -> ()
          n523 = global write "Robot Global Data.vi" "RightMotors"(w762) -> ()
        }
        frame #3 {
          n524 = global write "Robot Global Data.vi" "Gyro Rest?"(TRUE ("Gyro Rest?")) -> ()
          n525 = while {
            tunnel: w769 -> [w774]
            tunnel: w768 -> [w773]
            tunnel: [w772] -> w767
            tunnel: [w771] -> w766
            stop <- w780 stop-if-true
            n526 = global write "Robot Global Data.vi" "Gyro Rest?"(FALSE ("Gyro Rest?")) -> ()
            n527 = global read "Robot Global Data.vi" "LEFT SPEED VARIABLE"() -> (w776:dbl)
            n528 = global read "Robot Global Data.vi" "GyroAngle"() -> (w778:dbl)
            n529 = call <vilib>:"WPI_RobotDriveMotors.vi"("error in (no error)"=w773, "RightSpeed"=0.0 ("LeftSpeed"), "LeftSpeed"=w776, "RobotDriveDevRef"=w774) -> ("error out"=w771:errorcluster, "RobotDriveDevRef"=w772:T1)  [unwired: 5 in, 1 out]
            n530 = Equal?(x=w778, y=-40.0) -> (x = y?=w780:bool)
          }
        }
        frame #4 {
          n531 = global write "Robot Global Data.vi" "Gyro Rest?"(TRUE ("Gyro Rest?")) -> ()
          n532 = while {
            tunnel: w783 -> [w786]
            tunnel: w782 -> [w785]
            stop <- FALSE stop-if-true
            n533 = global read "Robot Global Data.vi" "GyroAngle"() -> (w788:dbl)
            n534 = global write "Robot Global Data.vi" "Gyro Rest?"(FALSE ("Gyro Rest?")) -> ()
            n535 = global read "Robot Global Data.vi" "X?"() -> (w789:dbl)
            n536 = call "vision sub.vi"("Gyro Angle"=w788, "X? Input"=w789) -> ("Right Motors"=w792:dbl, "Left Motors"=w793:dbl, "Nothing In Sight"=w791:bool)  [unwired: 7 in]
            n537 = global write "Robot Global Data.vi" "Vision Nothing In Sight"(w791) -> ()
            n538 = call <vilib>:"WPI_RobotDriveMotors.vi"("error in (no error)"=w785, "RightSpeed"=w792, "LeftSpeed"=w793, "RobotDriveDevRef"=w786) -> ("Motor Values"=w790:dbl[])  [unwired: 7 out]
            n539 = global write "Robot Global Data.vi" "RightMotors"(w792) -> ()
            n540 = global write "Robot Global Data.vi" "LeftMotors"(w793) -> ()
            n541 = global write "Robot Global Data.vi" "Motor Array"(w790) -> ()
          }
        }
      }
    }
    frame "Unleash The Hoppers" {
      n542 = flat-sequence {
        tunnel: [w807] -> w797
        tunnel: [w806] -> w796
        tunnel: w797 -> [w811]
        tunnel: w796 -> [w810]
        tunnel: [w809] -> w795
        tunnel: [w808] -> w794
        tunnel: w795 -> [w845]
        tunnel: w794 -> [w844]
        frame #0 {
          w799 = 0.0 ("TopLeftMotor")
          n543 = Wait (ms)(milliseconds to wait=u32 100) -> ()  [unwired: 1 out]
          n544 = global write "Robot Global Data.vi" "RightMotors"(w799) -> ()
          n545 = global write "Robot Global Data.vi" "LeftMotors"(w799) -> ()
          n546 = call <vilib>:"WPI_RobotDriveRefNum Registry Get.vi"("refnum name"="Motors") -> ("error out"=w807:errorcluster, "RobotDriveDevRef"=w800:T1)  [unwired: 9 in]
          n547 = call <vilib>:"WPI_RobotDriveMotors.vi"("RightSpeed"=w799, "LeftSpeed"=w799, "RobotDriveDevRef"=w800) -> ("Motor Values"=w798:dbl[], "RobotDriveDevRef"=w806:T1)  [unwired: 6 in, 1 out]
          n548 = global write "Robot Global Data.vi" "Motor Array"(w798) -> ()
          n549 = call <vilib>:"WPI_GyroRefNum Registry Get.vi"("refnum name"="My Gyro RefNum") -> ("error out"=w803:errorcluster, "GyroDevRef"=w804:T6)  [unwired: 9 in]
          n550 = call <vilib>:"WPI_GyroReset.vi"("error in"=w803, "GyroDevRef"=w804) -> ()  [unwired: 8 in, 2 out]
        }
        frame #1 {
          n551 = while {
            tunnel: w811 -> [w837]
            tunnel: w810 -> [w838]
            tunnel: [w836] -> w809
            tunnel: [w835] -> w808
            i -> [w813]
            stop <- w812 stop-if-true
            n552 = global read "Robot Global Data.vi" "GyroAngle"() -> (w827:dbl)
            n553 = global read "Robot Global Data.vi" "Autonomos Gyro forward SPEED VARIABLE"() -> (w817:dbl)
            n554 = expression code="(x/180.0)*pi" "degrees to radians"(w827) -> (w826:dbl)
            n555 = Negate(x=w826) -> (-x=w832:dbl)
            n556 = Sine(x=w832) -> (sin(x)=w821:dbl)
            n557 = Sine(x=w826) -> (sin(x)=w823:dbl)
            n558 = Add(x=w823, y=1.0 ("x")) -> (x+y=w822:dbl)
            n559 = Add(x=1.0, y=w821) -> (x+y=w820:dbl)
            n560 = Max & Min(x=w820, y=1.0) -> (min(x,y)=w830:dbl)  [unwired: 1 out]
            n561 = Max & Min(x=1.0, y=w822) -> (min(x,y)=w831:dbl)  [unwired: 1 out]
            n562 = global read "Robot Global Data.vi" "Autonoums Delay"() -> (w816:dbl)
            n563 = Multiply(x=w817, y=w830) -> (x*y=w829:dbl)
            n564 = Multiply(x=w817, y=w831) -> (x*y=w828:dbl)
            n565 = Negate(x=w829) -> (-x=w819:dbl)
            n566 = Negate(x=w828) -> (-x=w818:dbl)
            n567 = Add(x=w816, y=2000.0) -> (x+y=w815:dbl)
            n568 = call <vilib>:"WPI_RobotDriveMotors.vi"("error in (no error)"=w837, "RightSpeed"=w818, "LeftSpeed"=w819, "RobotDriveDevRef"=w838) -> ("error out"=w835:errorcluster, "Motor Values"=w839:dbl[], "RobotDriveDevRef"=w836:T1)  [unwired: 5 in]
            n569 = Equal?(x=w813, y=w815) -> (x = y?=w812:bool)
            n570 = global write "Robot Global Data.vi" "LeftMotors"(w819) -> ()
            n571 = global write "Robot Global Data.vi" "Motor Array"(w839) -> ()
            n572 = global write "Robot Global Data.vi" "RightMotors"(w818) -> ()
            n573 = Wait (ms)(milliseconds to wait=u32 1) -> ()  [unwired: 1 out]
          }
        }
        frame #2 {
          w842 = 0.0 ("LeftSpeed")
          n574 = call <vilib>:"WPI_RobotDriveMotors.vi"("error in (no error)"=w844, "RightSpeed"=w842, "LeftSpeed"=w842, "RobotDriveDevRef"=w845) -> ("Motor Values"=w841:dbl[])  [unwired: 5 in, 2 out]
          n575 = global write "Robot Global Data.vi" "LeftMotors"(w842) -> ()
          n576 = global write "Robot Global Data.vi" "Motor Array"(w841) -> ()
          n577 = global write "Robot Global Data.vi" "RightMotors"(w842) -> ()
          n578 = Wait (ms)(milliseconds to wait=u32 100) -> ()  [unwired: 1 out]
        }
      }
    }
  }
  n579 = while {
    stop <- FALSE stop-if-true
    n580 = call <vilib>:"WPI_DriverStationReport Robot Code State.vi"("Autonomous"=TRUE) -> ()  [unwired: 10 in, 1 out]
    n581 = Wait (ms)(milliseconds to wait=u32 20) -> ()  [unwired: 1 out]
  }
  n582 = global write "Robot Global Data.vi" "Autonomous Operating"(TRUE ("Autonomous Operating")) -> ()
